vi "ModelDiscrimination.vi"() -> ()   [LabVIEW 2015]
uses:
  <vilib>/Platform/TimedLoop/XDataNode/timing_clust.ctl
  <vilib>/Platform/TimedLoop/XDataNode/nitl_modes.ctl
  <vilib>/Platform/TimedLoop/XDataNode/wakeup.ctl
  <vilib>/DAQmx/read.llb/DAQmx Read (Analog DBL 1Chan 1Samp).vi
  <vilib>/DAQmx/read.llb/DAQmx Read (Analog 1D DBL NChan 1Samp).vi
  <vilib>/DAQmx/create/channels.llb/DAQmx Create Channel (AI-Voltage-Basic).vi
  <vilib>/Enthought/Python Integration Toolkit/api/Unpack Double.vi
  <vilib>/DAQmx/miscellaneous.llb/DAQmx Fill In Error Info.vi
  <vilib>/Platform/TimedLoop/XDataNode/XDataNode.xnode
  Program Files/neMESYS_SDK/neMESYS LabVIEW Kit/neMESYS LabVIEW Integration Kit.lvlib
  <vilib>/Platform/TimedLoop/XDataNode/XDNodeRunTimeDep.lvlib
  Conor/Temp CN7500/Omega CN7500/Omega CN7500.lvlib
  <vilib>/Enthought/Python Integration Toolkit/Python Integration Toolkit.lvlib
panel:
  out "Record filename, RecordAmbInitisileFactorial1":string
  out "HPLC file name, MBDoE2peakin1":string
  out "Exp 9":bool
  out "Temp 9":dbl
  out "Flow 9":dbl
  out "Conc 9":dbl
  out "X2 A 8":dbl
  out "X2 ref A 8":dbl
  out "X2 B 8":dbl
  out "X ref B 8":dbl
  out "C BAcid 8":dbl
  out "C EB 8":dbl
  out "Exp 8":bool
  out "Temp 8":dbl
  out "Flow 8":dbl
  out "Conc 8":dbl
  out "X2 A 7":dbl
  out "X2 ref A 7":dbl
  out "X2 B 7":dbl
  out "X ref B 7":dbl
  out "C BAcid 7":dbl
  out "C EB 7":dbl
  out "Exp 7":bool
  out "Temp 7":dbl
  out "Flow 7":dbl
  out "Conc 7":dbl
  out "X2 A 6":dbl
  out "X2 ref A 6":dbl
  out "X2 B 6":dbl
  out "X ref B 6":dbl
  out "C BAcid 6":dbl
  out "C EB 6":dbl
  out "Exp 6":bool
  out "Temp 6":dbl
  out "Flow 6":dbl
  out "Conc 6":dbl
  out "X2 A 5":dbl
  out "X2 ref A 5":dbl
  out "X2 B 5":dbl
  out "X ref B 5":dbl
  out "C BAcid 5":dbl
  out "C EB 5":dbl
  out "Exp 5":bool
  out "Temp 5":dbl
  out "Flow 5":dbl
  out "Conc 5":dbl
  out "X2 A 4":dbl
  out "X2 ref A 4":dbl
  out "X2 B 4":dbl
  out "X ref B 4":dbl
  out "C BAcid 4":dbl
  out "C EB 4":dbl
  out "Exp 4":bool
  out "Temp 4":dbl
  out "Flow 4":dbl
  out "Conc 4":dbl
  out "X2 A 3":dbl
  out "X2 ref A 3":dbl
  out "X2 B 3":dbl
  out "X ref B 3":dbl
  out "C BAcid 3":dbl
  out "C EB 3":dbl
  out "Exp 3":bool
  out "Temp 3":dbl
  out "Flow 3":dbl
  out "Conc 3":dbl
  out "X2 A 2":dbl
  out "X2 ref A 2":dbl
  out "X2 B 2":dbl
  out "X ref B 2":dbl
  out "C BAcid 2":dbl
  out "C EB 2":dbl
  in  "Cat Mass (0.096 g)":dbl
  in  "Cat Diameter (825 um)":dbl
  out "X2 A 1":dbl
  out "X2 ref A 1":dbl
  out "X2 B 1":dbl
  out "X ref B 1":dbl
  out "Exp 1":bool
  out "C EB 1":dbl
  out "C BAcid 1":dbl
  out "Liquid Inlet Pressure (bar g)":dbl
  in  "Liquid P sensor Terminal Configuration":i32(ring)=-1 items=["default"=-1, "RSE"=10083, "NRSE"=10078, "Differential"=10106, "Pseudodifferential"=12529]
  in  "Liquid P sensor Physical Channel":tag="Dev1/ai0"
  out "Exp 2":bool
  out "Exp 0":bool
  out "Conc 1":dbl
  out "Flow 1":dbl
  out "Temp 1":dbl
  out "Conc 2":dbl
  out "Flow 2":dbl
  out "Temp 2":dbl
  out "X2 A":dbl
  out "X2 ref  A":dbl
  out "X2 B":dbl
  out "X2 ref B":dbl
  out "Desired Conc Not Possible":bool
  in  "Safety or Emergency Syringe Control":bool
  out "Feed Concentration (M)":dbl
  out "Total Flowrate (uL/min)":dbl
  out "Gas Back Pressure (barg)":dbl
  in  "Shut down in empty?\nLeft off, right on":bool
  in  "Clear":bool
  out "Safety Shut Down Pressure (barg)":dbl
  out "Calculated Pressure":dbl[](graph)
  out "Safety Shut Down Temp":dbl
  out "Actual Temp (oC)":dbl
  out "Temperature":dynamicdata(graph)
  out "Temp Set Point (oC)":dbl
  in  "Temp 0":dbl
  in  "Update Temperature Set Point":bool
  in  "Automated Experiments or Direct Control":bool
  in  "Set Point (oC)":dbl
  out "loop ind":dbl
  in  "Stop everything":bool
  in  "Skip Exp":bool
  in  "Minutes between Exp":dbl min=0.0 step=0.05
  in  "Refill 4":bool
  in  "Refill 3":bool
  in  "Refill 2":bool
  in  "Refill 1":bool
  in  "Empty 4":bool
  in  "Empty 3":bool
  in  "Empty 2":bool
  in  "Empty 1":bool
  in  "Calibrate 4":bool
  in  "Calibrate 3":bool
  in  "Calibrate 2":bool
  in  "Calibrate 1":bool
  in  "Stop Dose 4":bool
  in  "Stop Dose 3":bool
  in  "Stop Dose 2":bool
  in  "Stop Dose 1":bool
  in  "Flow 0":dbl
  in  "Conc 0":dbl
  in  "Generate Flow":bool
  in  "Set Flowrate 1":dbl
  in  "Set Flowrate 2":dbl
  in  "Set Flowrate 3":dbl
  in  "Set Flowrate 4":dbl
  in  "High Conc":dbl min=0.0 max=2.0
  in  "Low Conc":dbl min=0.0 max=2.0
  out "Syringe Level 4":dbl(slide) scale=0.0..5500.0
  out "Syringe Level 3":dbl(slide) scale=0.0..5500.0
  out "Syringe Level 2":dbl(slide) scale=0.0..5500.0
  out "Syringe Level 1":dbl(slide) scale=0.0..5500.0
  out "Flowrate 4 High":dbl
  out "Flowrate 3 High":dbl
  out "Flowrate 2 Low":dbl
  out "Flowrate 1 Low":dbl
  # "Pre Planned Experiments"
  # "Conducted Experiments Set Points"
  # "Safety (start and end)"
  # "Current Conditions"
  # "(uL/min)"
  # "Coerced to nearest possible"
  # "Experimental Info"
  # "This code only does Automated \nDirect control just sets all variables to 0"
  # "Direct Control"
  # "Unit of Gas Flow NmL/min"
  # "Emergency Syringe Control Below"
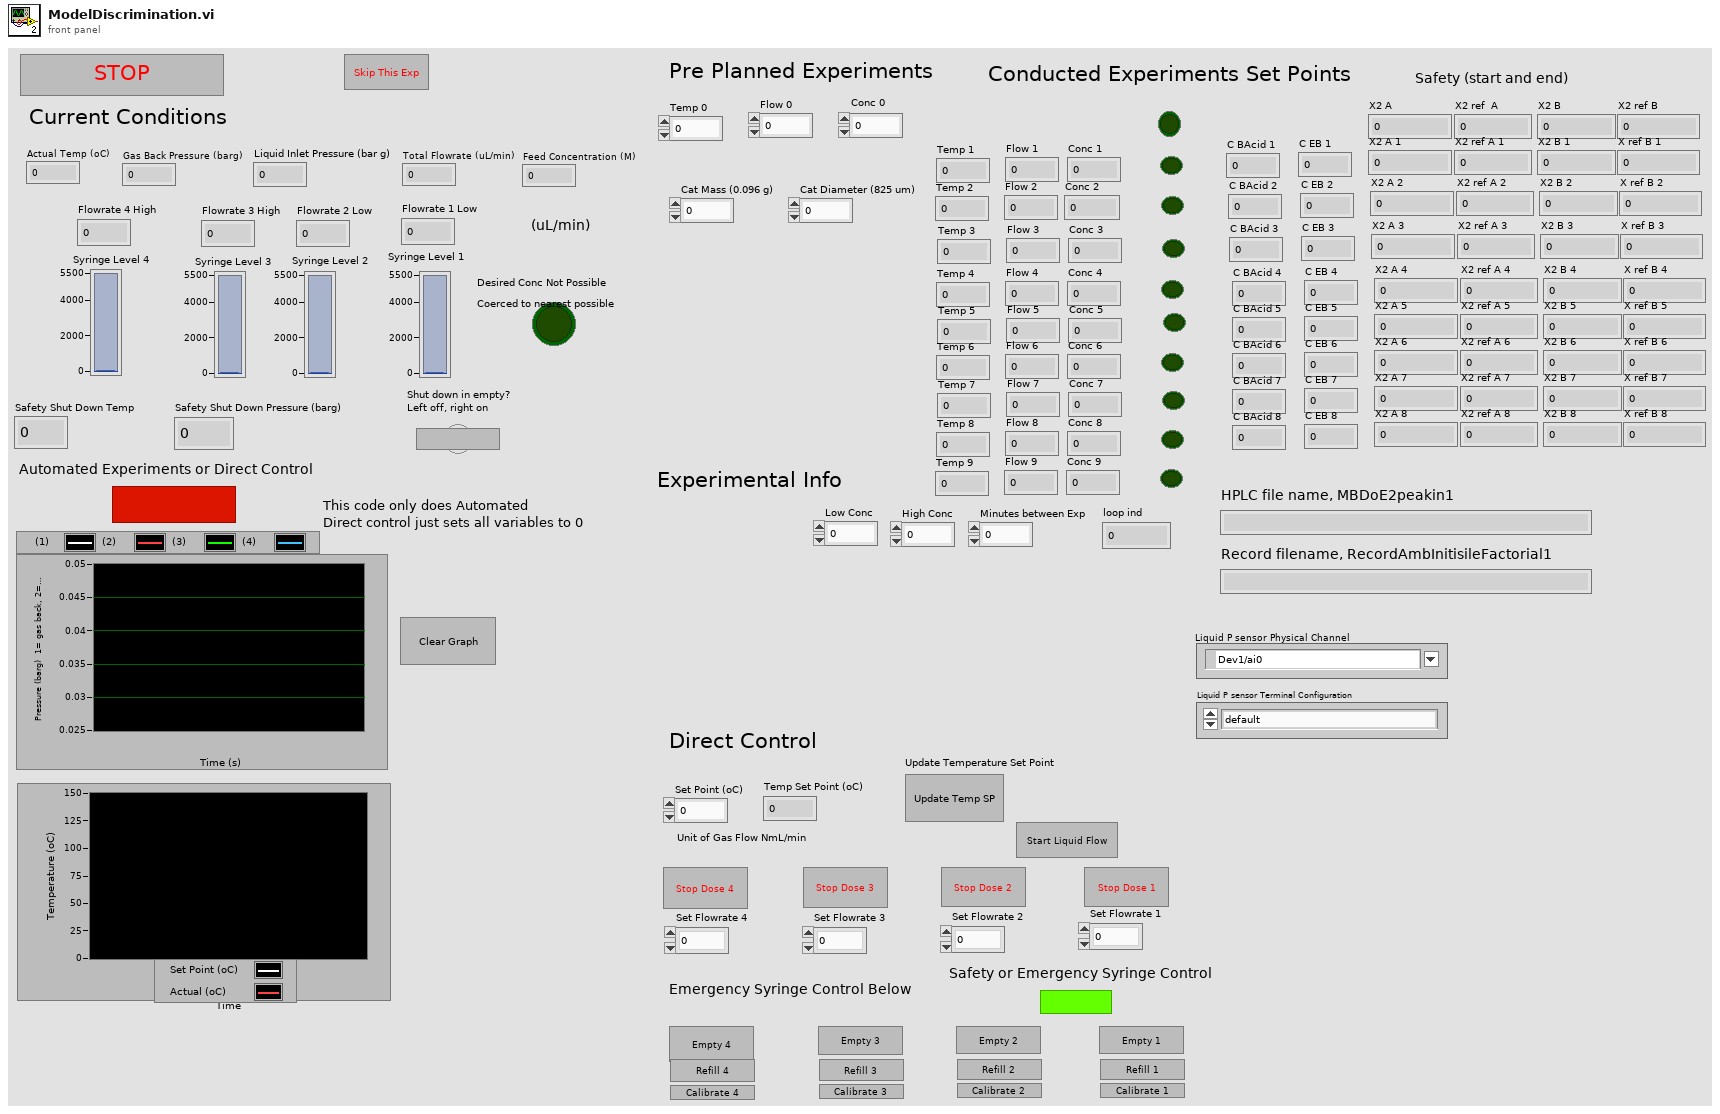
[diagram p1: front panel]
types:
  T1 = typedef "XDNodeRunTimeDep.lvlib/timing_clust.ctl" = cluster{"Expected End [f-1]":u64, "Actual End [f-1]":u64, "Finished Late? [f-1]":bool, "Expected End [i-1]":u64, "Actual End [i-1]":u64, "Finished Late? [i-1]":bool, "Expected Start [i]":u64, "Actual Start [i]":u64, "Expected Start [f]":u64, "Actual Start [f]":u64, "Source Name":string, "Structure Name":string, "Period":i64, "Deadline":i64, "Offset":i64, "Start":i64, "Priority":i32, "Timeout":i32, "Mode":T2, "Wakeup Reason":T3, "Error":errorcluster, "Source Type":string, "Secondary Source Type":string, "Global End Time":u64, "Global Start Time":u64, "Frame Duration":u64, "Iteration Duration":u64, "Assigned CPU":i32, "I/O Scan Engine Mode":u32}
  T2 = typedef "XDNodeRunTimeDep.lvlib/nitl_modes.ctl" = enum32{"No Change", "Process missed periods, maintain original phase", "Discard missed periods, maintain original phase", "Process missed periods, ignore original phase", "Discard missed periods, ignore original phase"}
  T3 = typedef "XDNodeRunTimeDep.lvlib/wakeup.ctl" = enum32{"Normal", "Aborted", "Asynchronous wakeup", "Timing source error", "Timed loop error", "Timeout"}
  T4 = typedef "Python Integration Toolkit.lvlib/Session ID.ctl" = u64
  T5 = typedef "Python Integration Toolkit.lvlib/Python Objects.ctl" = variant
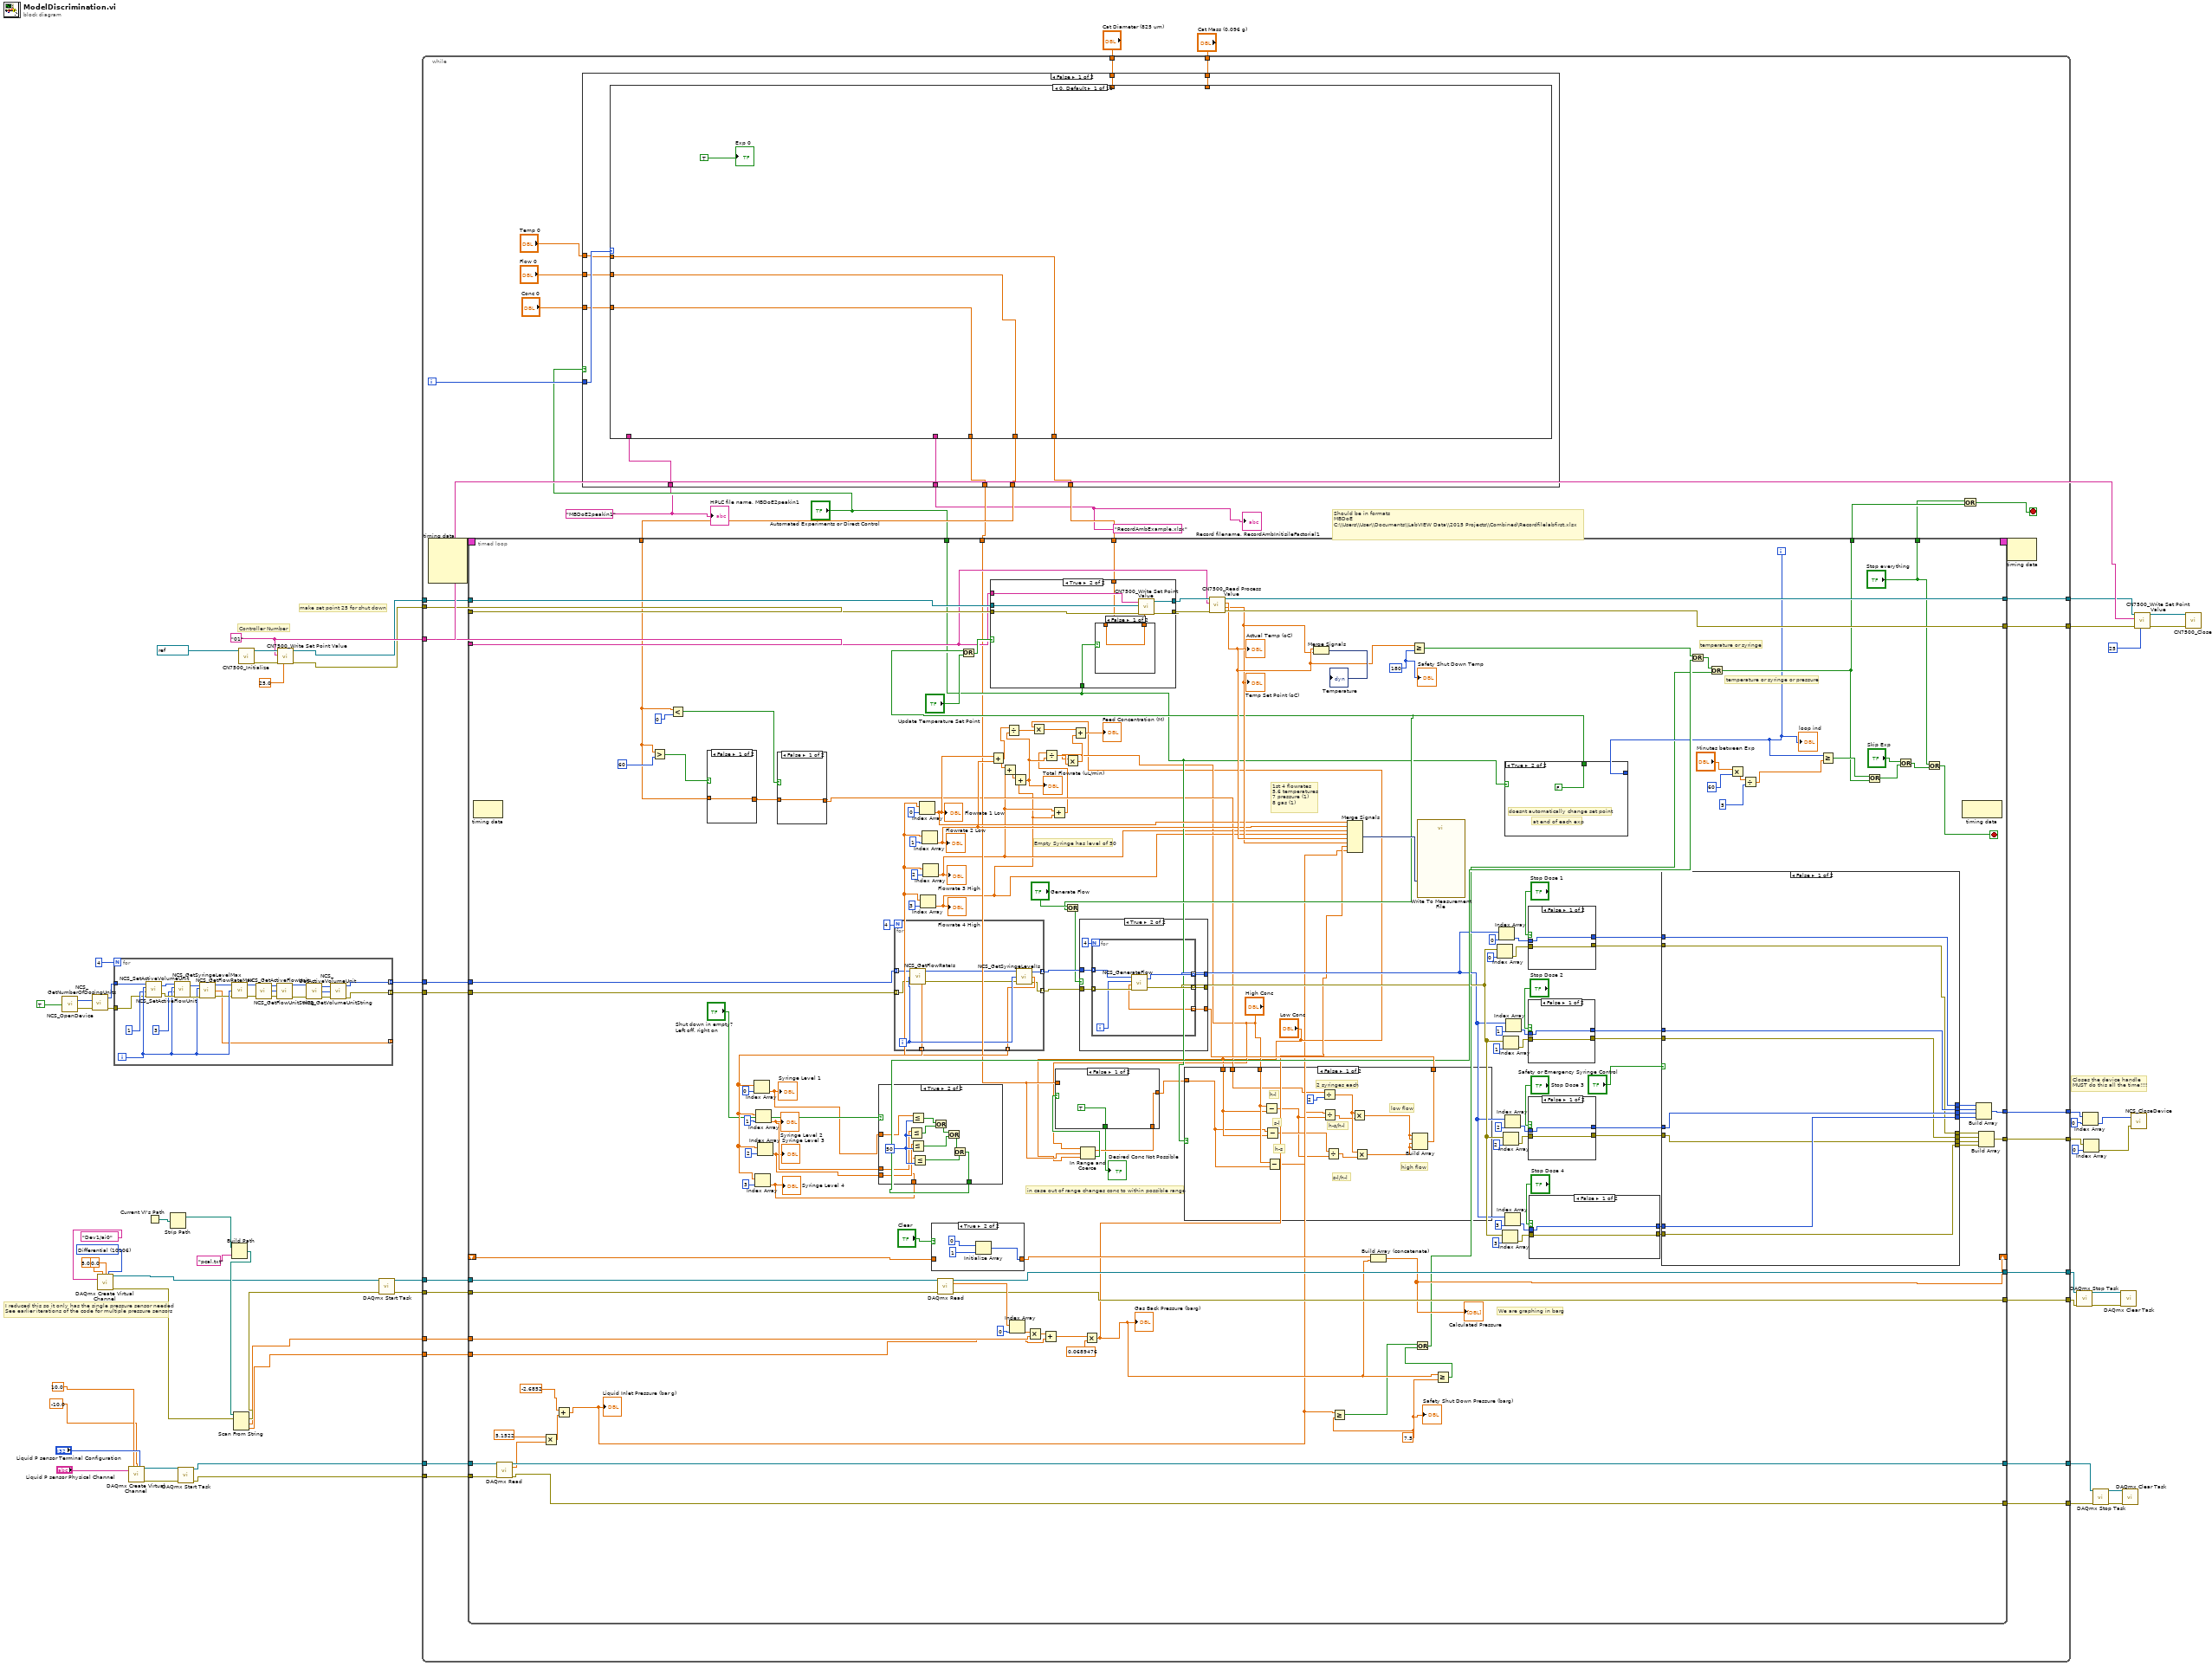
[diagram p0: block diagram]
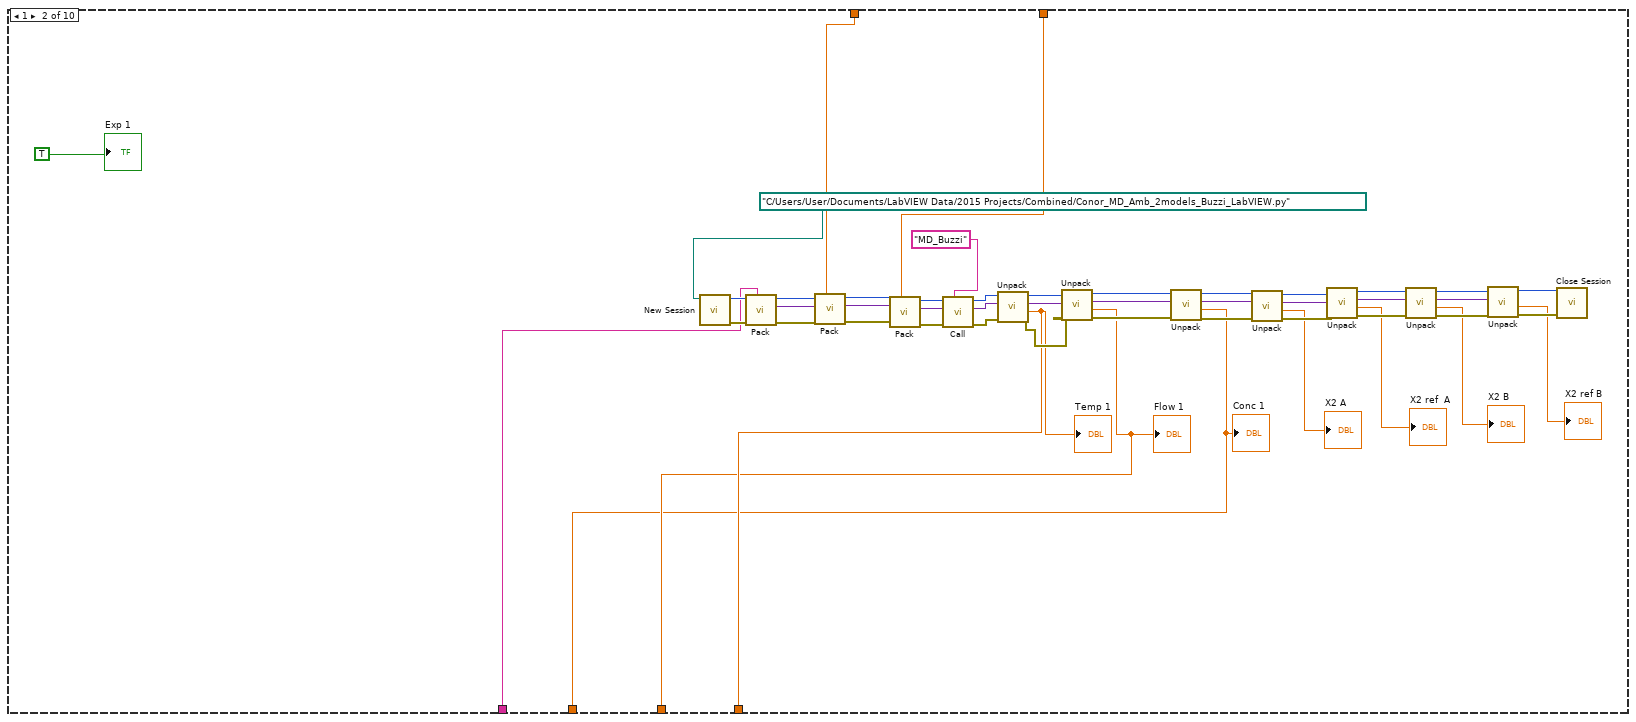
[diagram p2: hidden frame]
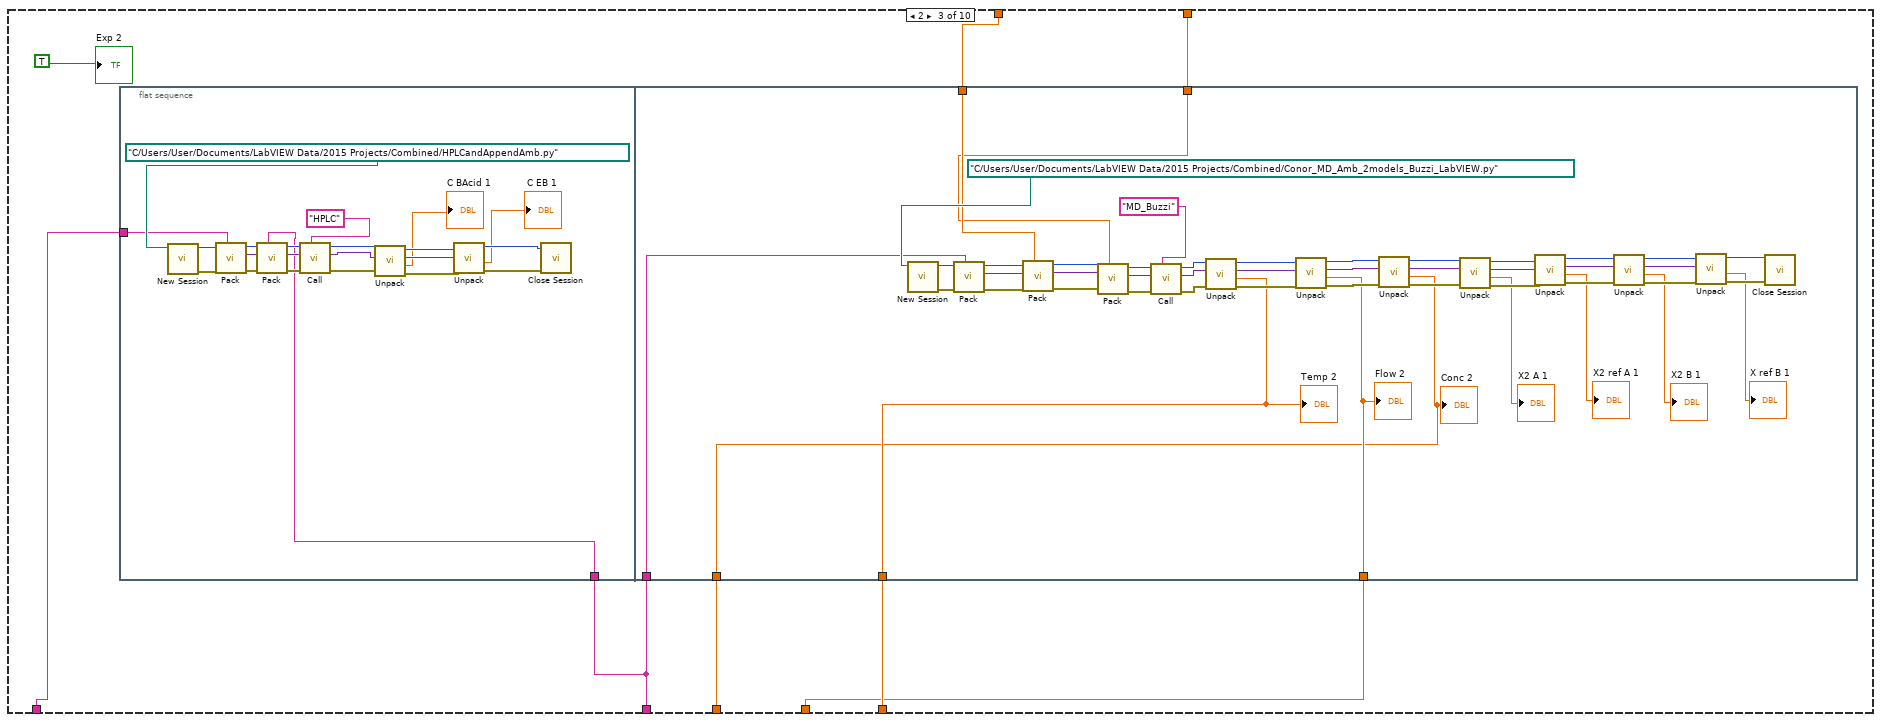
[diagram p3: hidden frame]
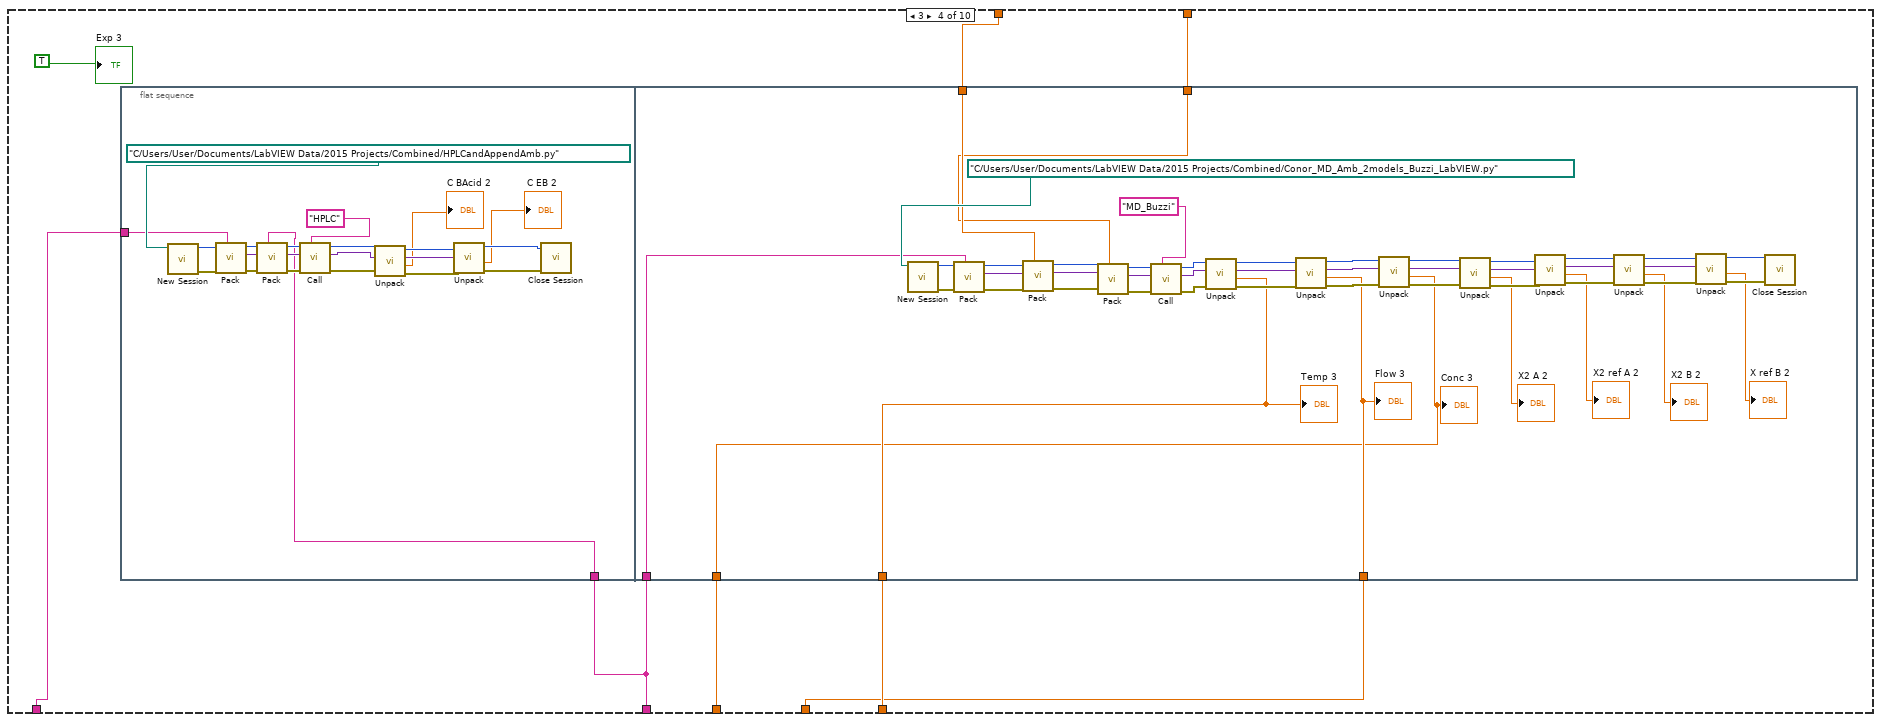
[diagram p4: hidden frame]
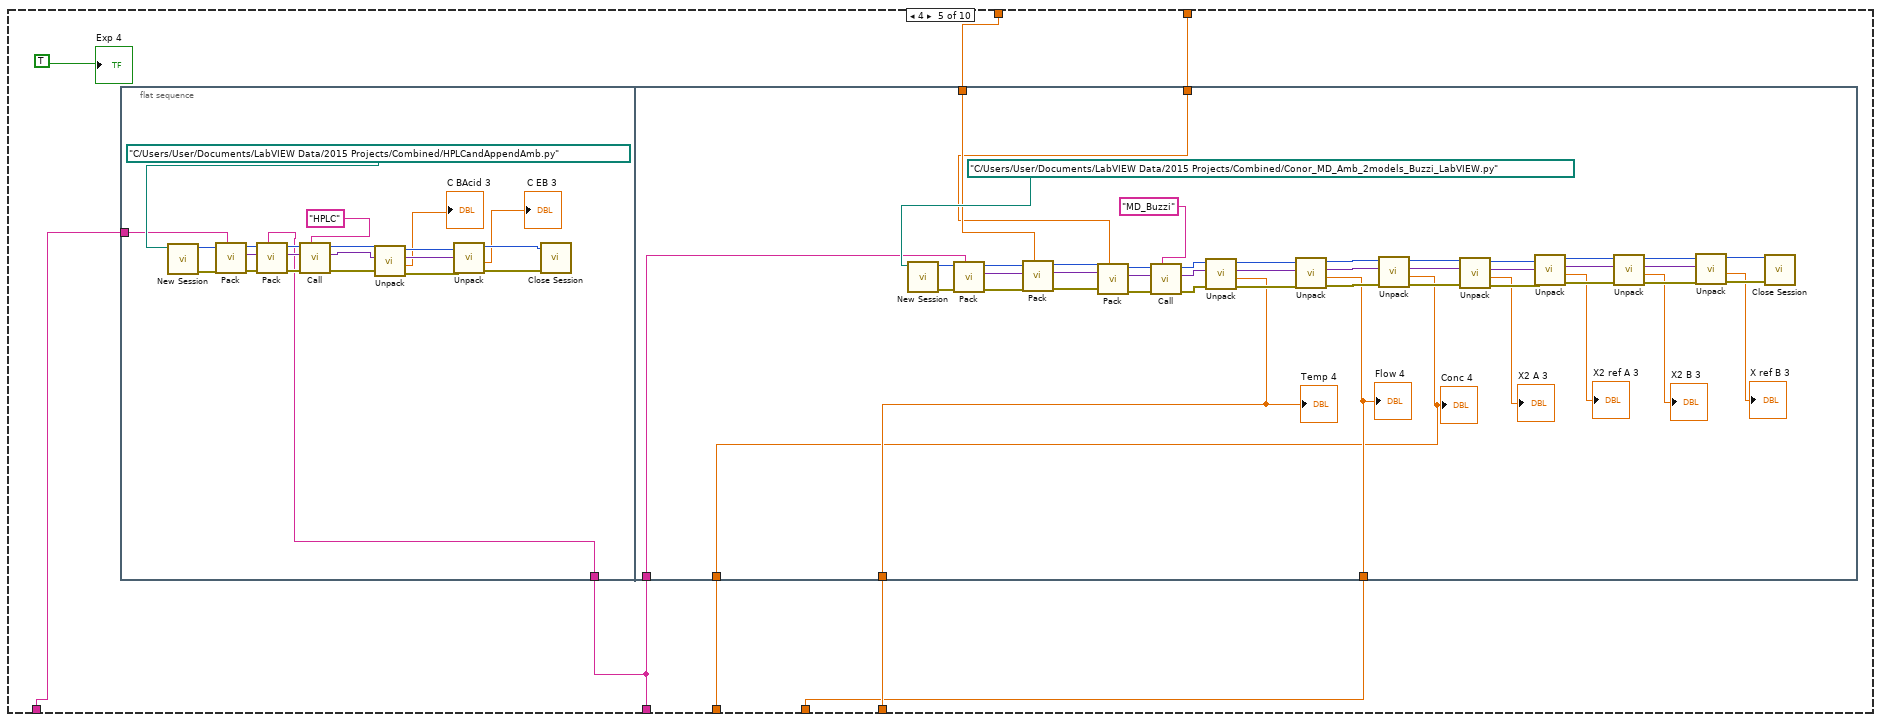
[diagram p5: hidden frame]
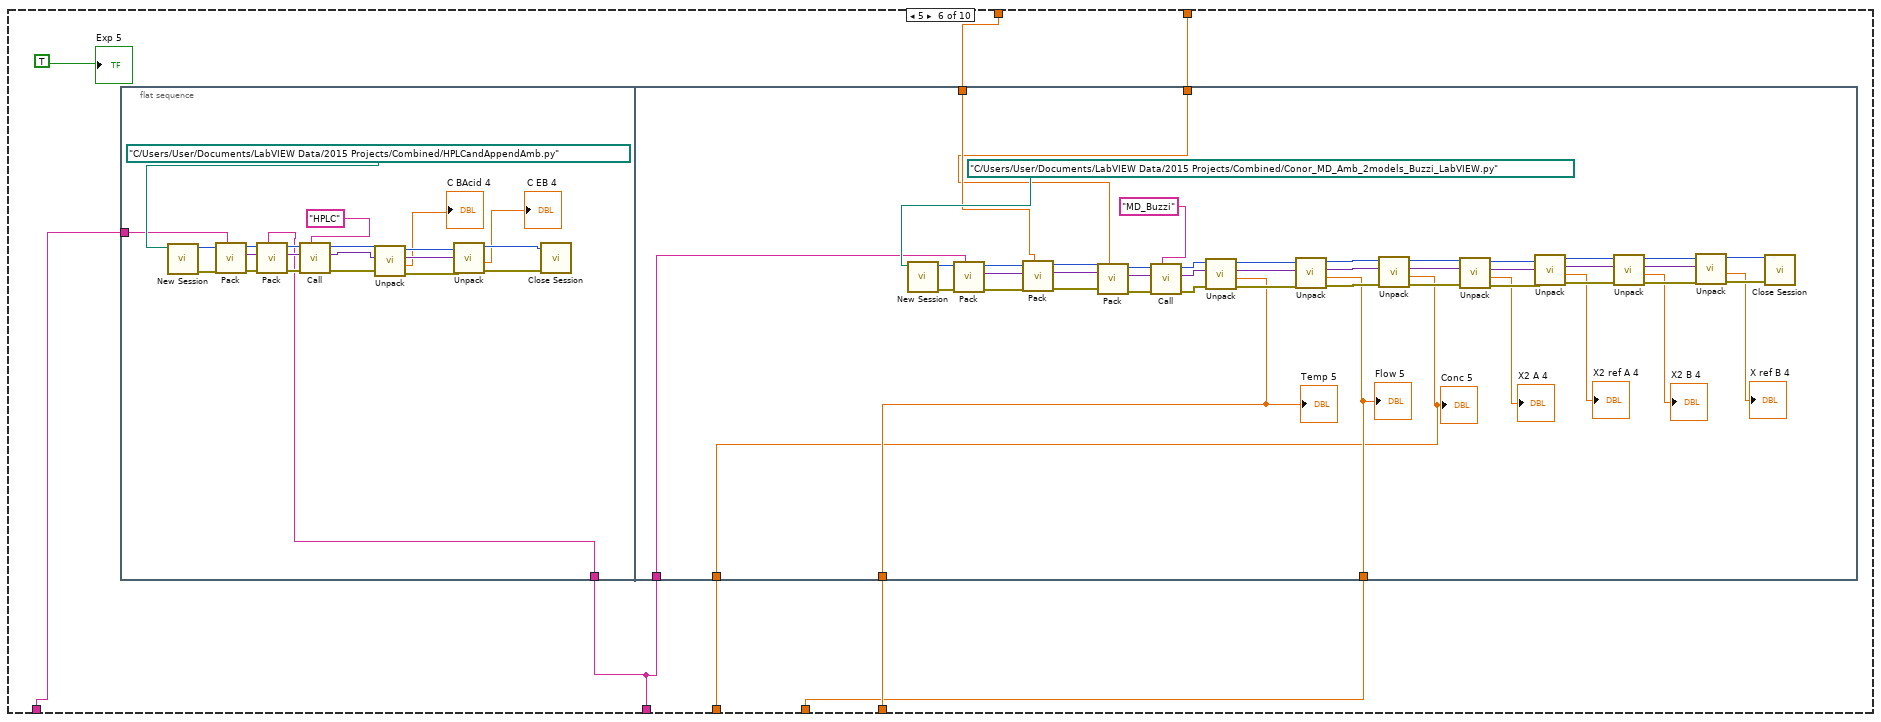
[diagram p6: hidden frame]
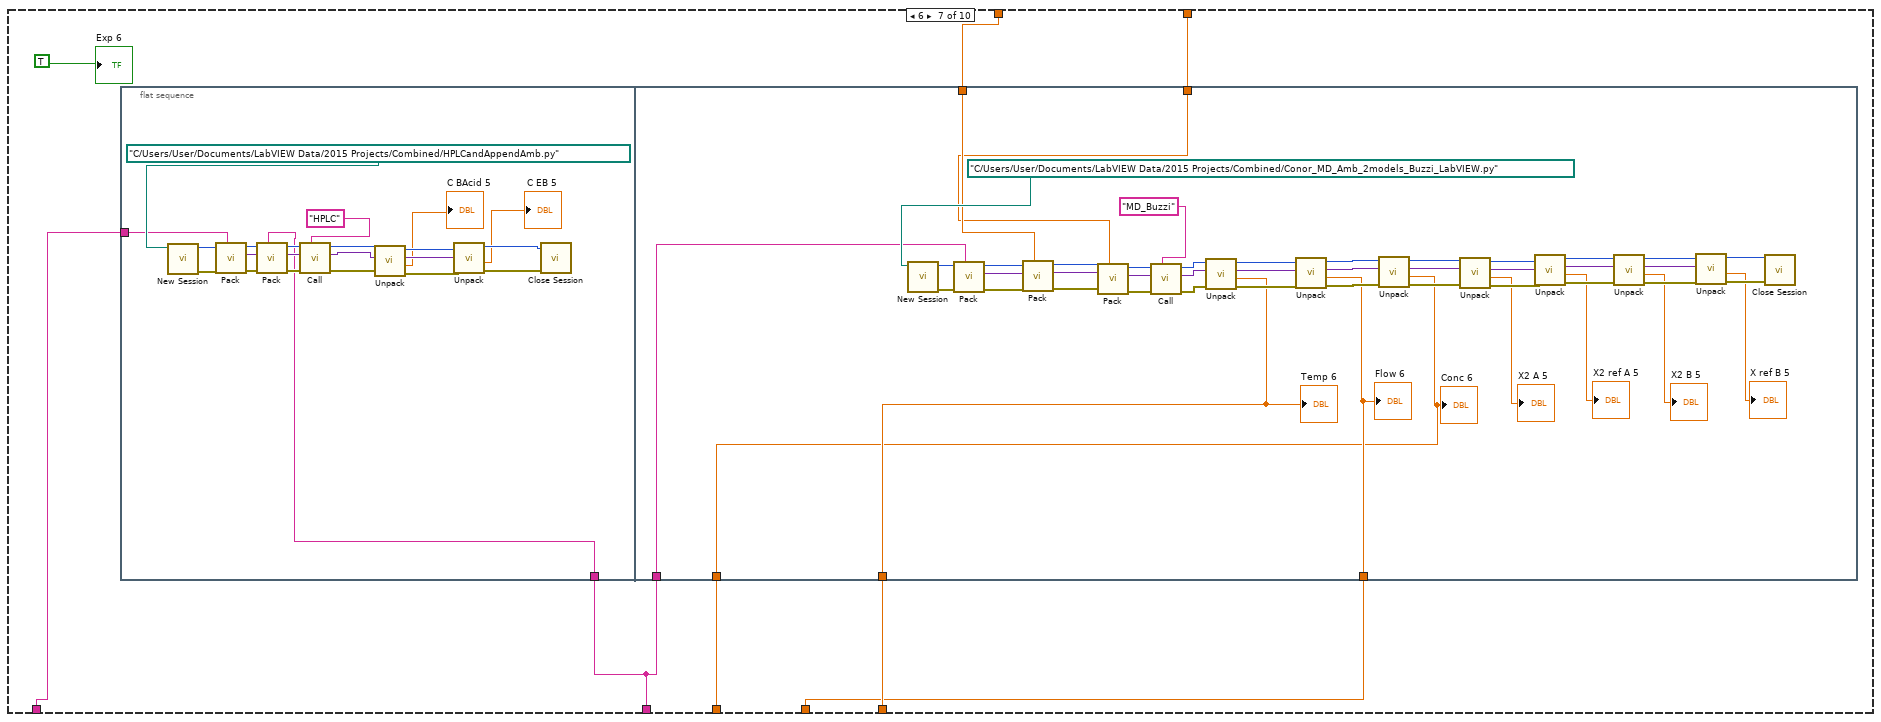
[diagram p7: hidden frame]
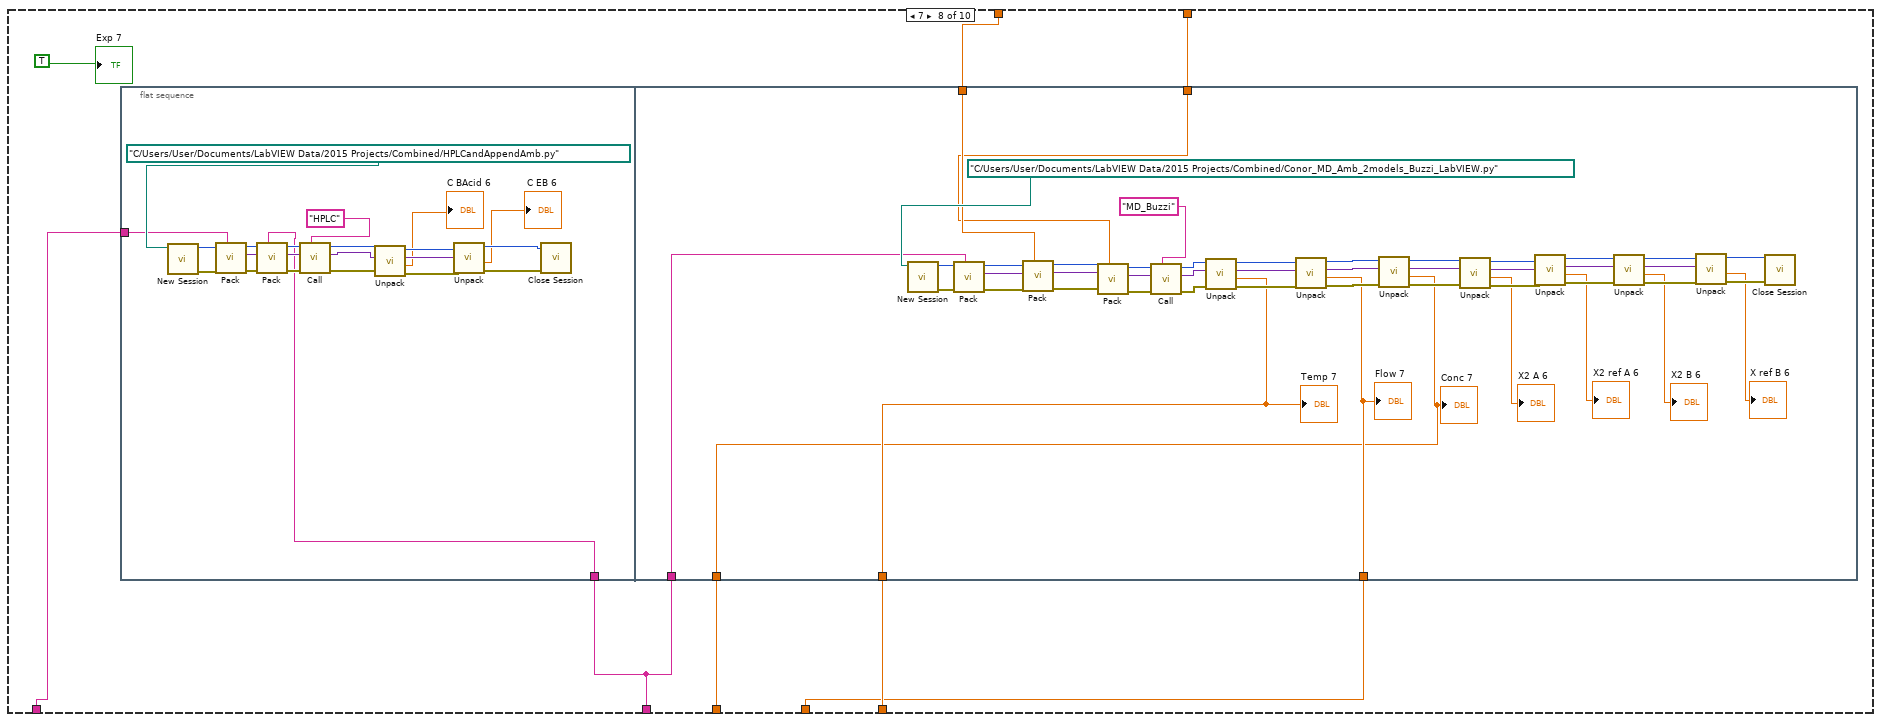
[diagram p8: hidden frame]
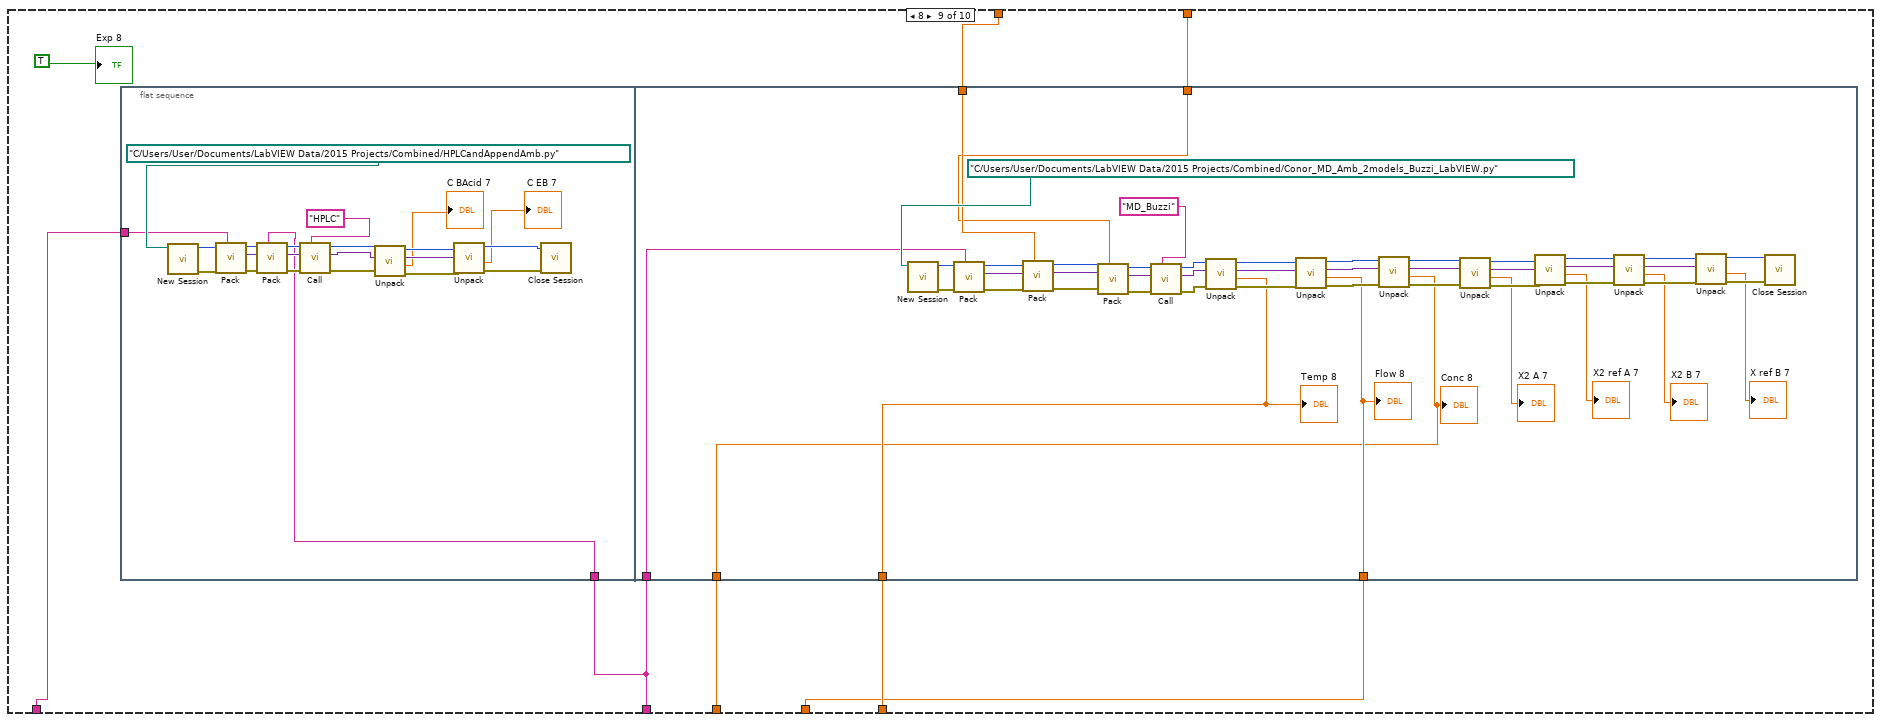
[diagram p9: hidden frame]
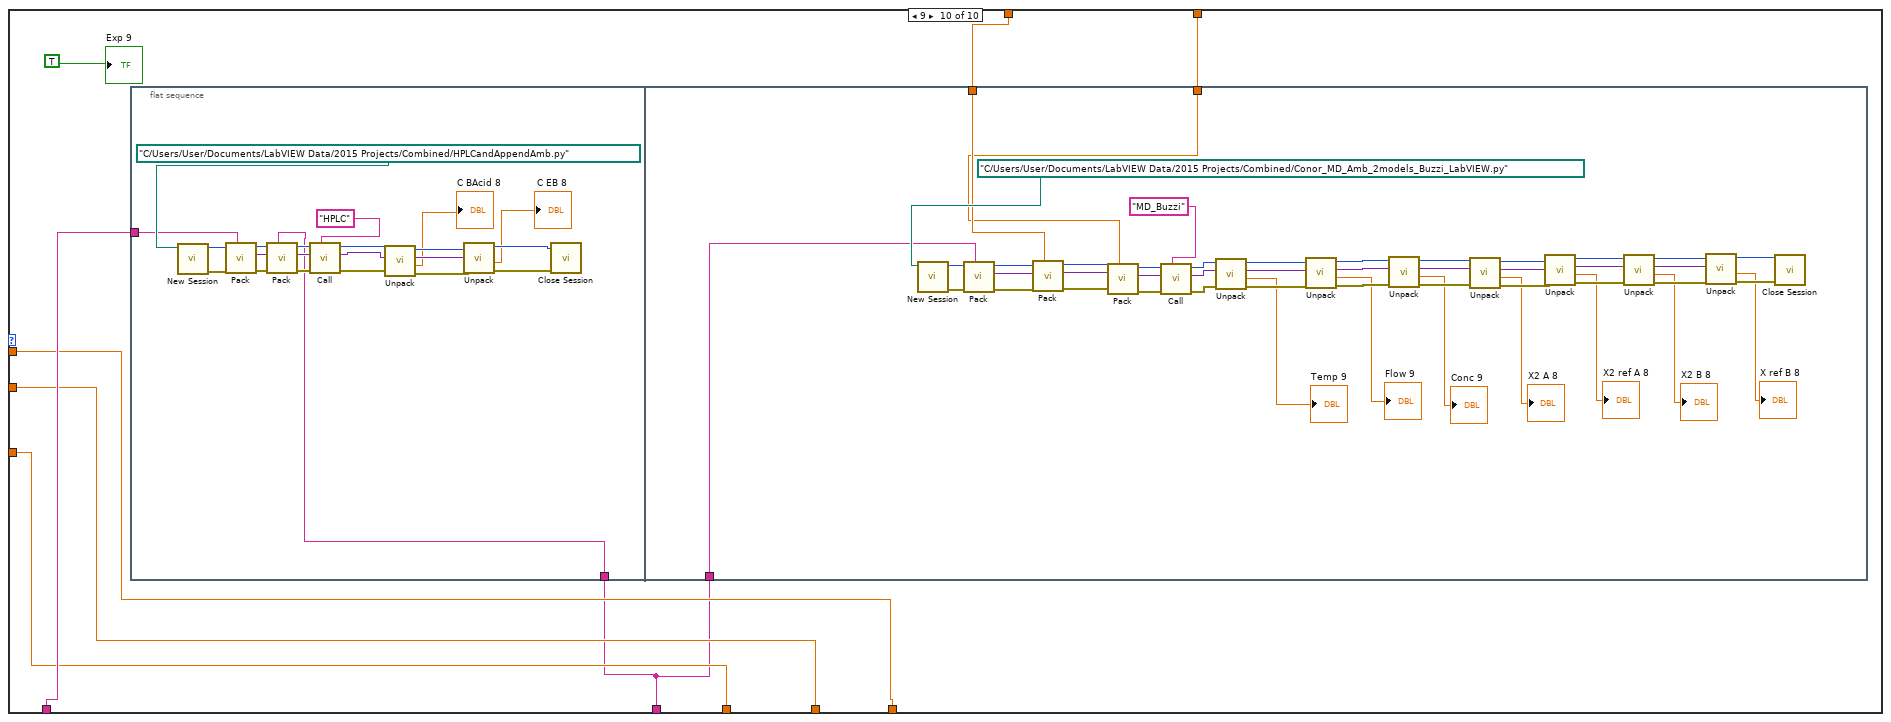
[diagram p10: hidden frame]
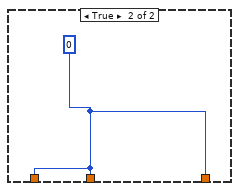
[diagram p11: hidden frame]
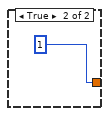
[diagram p12: hidden frame]
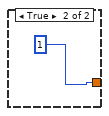
[diagram p13: hidden frame]
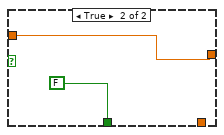
[diagram p14: hidden frame]
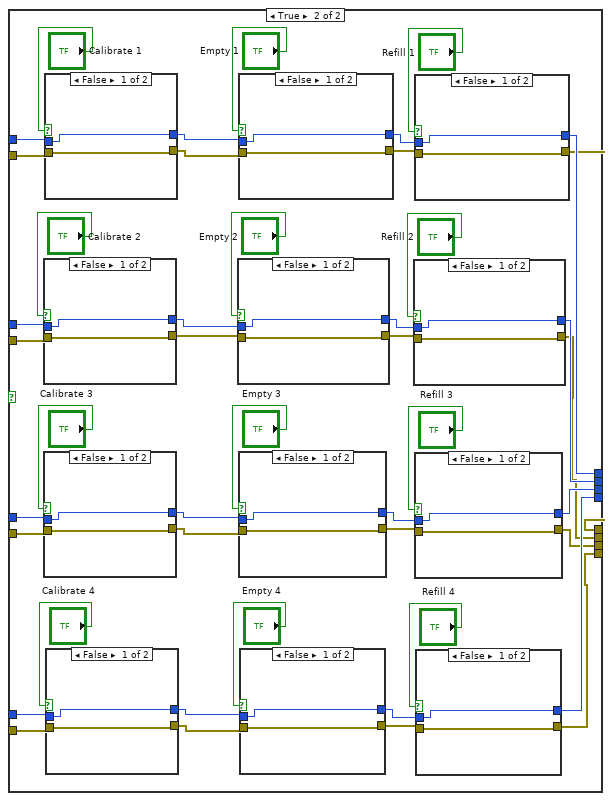
[diagram p15: hidden frame]
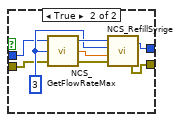
[diagram p16: hidden frame]
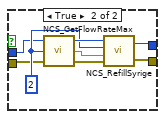
[diagram p17: hidden frame]
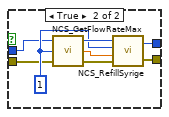
[diagram p18: hidden frame]
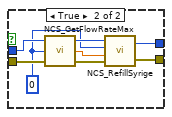
[diagram p19: hidden frame]
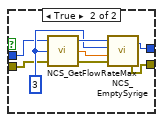
[diagram p20: hidden frame]
diagram:
  w31 = 10106 items=["default"=-1, "RSE"=10083, "NRSE"=10078, "Differential"=10106, "Pseudodifferential"=12529] ("input terminal configuration")
  w38 = "01" ("Controller Number")
  # "I reduced this so it only has the single pressure sensor needed\nSee earlier iterations of the code for multiple pressure sensors"
  # "make set point 25 for shut down"
  # "Controller Number"
  # "Closes the device handle \nMUST do this all the time!!!!"
  n1 = call "NCS_OpenDevice.vi"("show status window"=TRUE) -> ("device handle"=w57:u32, "error out"=w56:errorcluster)
  n2 = call "NCS_GetNumberOfDosingUnits.vi"("device handle in"=w57, "error in (no error)"=w56) -> ("device handle out"=w54:u32, "error out"=w55:errorcluster)  [unwired: 1 out]
  n3 = call-poly <vilib>:"DAQmx Create Virtual Channel.vi"("maximum value"=5.0, "minimum value"=0.0, "input terminal configuration"=w31, "physical channels"=tag "Dev1/ai0") -> ("task out"=w15:refnum<k21>, "error out"=w16:errorcluster)  [unwired: 10 in]
  n4 = for {
    N: 4 -> [_]
    tunnel: [w63] -> w53 mode=indexing
    tunnel: [w62] -> w52 mode=indexing
    tunnel: [w76] -> _ mode=indexing
    tunnel: w55 -> [w61]
    tunnel: w54 -> [w60]
    i -> [w79]
    n5 = call "NCS_SetActiveVolumeUnit.vi"("error in (no error)"=w61, "active volume unit"=1, "dosingunit"=w79, "device handle in"=w60) -> ("error out"=w82:errorcluster, "device handle out"=w83:u32)
    n6 = call "NCS_SetActiveFlowUnit.vi"("error in (no error)"=w82, "active flow unit"=3, "dosingunit"=w79, "device handle in"=w83) -> ("error out"=w80:errorcluster, "device handle out"=w81:u32)
    n7 = call "NCS_GetSyringeLevelMax.vi"("error in (no error)"=w80, "dosingunit"=w79, "device handle in"=w81) -> ("error out"=w77:errorcluster, "syringe level max"=w76:dbl, "device handle out"=w78:u32)  [unwired: 1 out]
    n8 = call "NCS_GetFlowRateMax.vi"("error in (no error)"=w77, "dosingunit"=w79, "device handle in"=w78) -> ("error out"=w64:errorcluster, "device handle out"=w65:u32)  [unwired: 1 out]
    n9 = call "NCS_GetActiveFlowUnit.vi"("error in (no error)"=w64, "device handle in"=w65) -> ("error out"=w72:errorcluster, "active flow unit"=w71:u8, "device handle out"=w73:u32)  [unwired: 1 in]
    n10 = call "NCS_GetFlowUnitString.vi"("device handle in"=w73, "flow unit id"=w71, "error in (no error)"=w72) -> ("device handle out"=w68:u32, "error out"=w67:errorcluster)  [unwired: 2 out]
    n11 = call "NCS_GetActiveVolumeUnit.vi"("error in (no error)"=w67, "device handle in"=w68) -> ("error out"=w69:errorcluster, "active volume unit"=w70:u8, "device handle out"=w66:u32)  [unwired: 1 in]
    n12 = call "NCS_GetVolumeUnitString.vi"("device handle in"=w66, "volume unit id"=w70, "error in (no error)"=w69) -> ("device handle out"=w63:u32, "error out"=w62:errorcluster)  [unwired: 2 out]
  }
  n13 = call-poly <vilib>:"DAQmx Create Virtual Channel.vi"("maximum value"=10.0, "minimum value"=-10.0 ("maximum value"), "input terminal configuration"="Liquid P sensor Terminal Configuration", "physical channels"="Liquid P sensor Physical Channel") -> ("task out"=w11:refnum<k21>, "error out"=w12:errorcluster)  [unwired: 10 in]
  n14 = Current VI's Path() -> (path=w29:path)
  n15 = Strip Path(path=w29) -> (stripped path=w27:path)  [unwired: 1 out]
  n16 = call <vilib>:"DAQmx Start Task.vi"("task/channels in"=w11, "error in"=w12) -> ("task out"=w10:refnum<k21>, "error out"=w9:errorcluster)  [unwired: 12 in]
  n17 = Build Path(base path=w27, name or relative path="pcal.txt") -> (appended path=w28:path)
  n18 = Scan From String(w28, w16) -> (w25:errorcluster, output 1=w22:dbl, output 2=w21:dbl)  [unwired: 3 in, 1 out]
  n19 = call "CN7500_Initialize.vi"("VISA resource name"=refnum<visa-resource-name> "COM8") -> ("error out"=w44:errorcluster, "VISA resource name out"=w45:refnum<visa-resource-name>)  [unwired: 9 in]
  n20 = call "CN7500_Write Set Point Value.vi"("Target Set Point Value"=25.0, "error in (no error)"=w44, "Controller Number"=w38, "VISA In"=w45) -> ("error out"=w36:errorcluster, "VISA Out"=w37:refnum<visa-resource-name>)  [unwired: 6 in]
  n21 = call <vilib>:"DAQmx Start Task.vi"("task/channels in"=w15, "error in"=w25) -> ("task out"=w24:refnum<k21>, "error out"=w23:errorcluster)  [unwired: 12 in]
  n22 = while {
    tunnel: w53 -> [w119]
    tunnel: w52 -> [w118]
    tunnel: [w117] -> w47
    tunnel: [w116] -> w46
    tunnel: w38 -> [w113]
    tunnel: w37 -> [w112]
    tunnel: w36 -> [w111]
    tunnel: [w110] -> w35
    tunnel: [w109] -> w34
    tunnel: w24 -> [w107]
    tunnel: w23 -> [w106]
    tunnel: w22 -> [w105]
    tunnel: w21 -> [w104]
    tunnel: [w103] -> w18
    tunnel: [w102] -> w17
    tunnel: w10 -> [w91]
    tunnel: w9 -> [w90]
    tunnel: [w89] -> w7
    tunnel: [w88] -> w5
    tunnel: "Cat Diameter (825 um)" -> [w87]
    tunnel: "Cat Mass (0.096 g)" -> [w86]
    i -> [w96]
    stop <- w101 stop-if-true
    w84 = "RecordAmbExample.xlsx" ("Result file name must end with .xlsx")
    w85 = "MBDoE2peakin1" ("HPLC file Name, dont need extension")
    # "Should be in formats \nMBDoE\nC:\\\\Users\\\\User\\\\Documents\\\\LabVIEW Data\\\\2015 Projects\\\\Combined\\Recordfilelabfirst.xlsx"
    n23 = node-c288() -> (w115:T1)  [unwired: 4 in]
    n24 = case shown="False" "Automated Experiments or Direct Control" {
      tunnel: [w127 w790] -> w99
      tunnel: [w125 w790] -> w98
      tunnel: [w129 w790] -> w97
      tunnel: w96 -> [w130 _]
      tunnel: "Conc 0" -> [w128 _]
      tunnel: "Flow 0" -> [w124 _]
      tunnel: "Temp 0" -> [w126 _]
      tunnel: w85 -> [w122 _]
      tunnel: w84 -> [w123 _]
      tunnel: w87 -> [w121 _]
      tunnel: w86 -> [w120 _]
      frame False {
        n25 = case shown="0, Default" w130 {
          tunnel: [w132 w135 w185 w261 w337 w413 w489 w565 w641 w717] -> w129
          tunnel: w128 -> [w132 _ _ _ _ _ _ _ _ w717]
          tunnel: [w134 w137 w187 w263 w339 w415 w491 w567 w643 w719] -> w127
          tunnel: w126 -> [w134 _ _ _ _ _ _ _ _ w719]
          tunnel: [w133 w136 w186 w262 w338 w414 w490 w566 w642 w718] -> w125
          tunnel: w124 -> [w133 _ _ _ _ _ _ _ _ w718]
          tunnel: w123 -> [_ w142 w184 w260 w336 w412 w488 w564 w640 w716]
          tunnel: w122 -> [_ _ w188 w264 w340 w416 w492 w568 w644 w720]
          tunnel: w121 -> [_ w145 w183 w259 w335 w411 w487 w563 w639 w715]
          tunnel: w120 -> [_ w144 w182 w258 w334 w410 w486 w562 w638 w714]
          frame 0, Default {
            "Exp 0" <- TRUE
          }
          frame 1 {
            n26 = call <vilib>:"New Session.vi"("Path to Python Module (.py File)"=path "C:/Users/User/Documents/LabVIEW Data/2015 Projects/Combined/Conor_MD_Amb_2models_Buzzi_LabVIEW.py") -> ("error out"=w173:errorcluster, "Session ID out"=w172:T4)  [unwired: 9 in]
            n27 = call <vilib>:"Pack.vi"("Argument"=w142, "error in (no error)"=w173, "Session ID"=w172) -> ("error out"=w166:errorcluster, "Python Object References Out"=w167:T5, "Session ID out"=w168:T4)  [unwired: 6 in]
            n28 = call <vilib>:"Pack.vi"("Argument"=w145, "error in (no error)"=w166, "Python Object References In"=w167, "Session ID"=w168) -> ("error out"=w148:errorcluster, "Python Object References Out"=w150:T5, "Session ID out"=w149:T4)  [unwired: 5 in]
            n29 = call <vilib>:"Pack.vi"("Argument"=w144, "error in (no error)"=w148, "Python Object References In"=w150, "Session ID"=w149) -> ("error out"=w151:errorcluster, "Python Object References Out"=w152:T5, "Session ID out"=w153:T4)  [unwired: 5 in]
            n30 = call <vilib>:"Call.vi"("Function or Method Name"="MD_Buzzi", "error in (no error)"=w151, "Python Object References In"=w152, "Session ID"=w153) -> ("error out"=w159:errorcluster, "Python Object References Out"=w162:T5, "Session ID out"=w165:T4)  [unwired: 5 in]
            n31 = call-poly <vilib>:"Unpack.vi"("error in (no error)"=w159, "Python Object References In"=w162, "Session ID"=w165) -> ("error out"=w158:errorcluster, "Value"=w137:dbl, "Python Object References Out"=w161:T5, "Session ID out"=w164:T4)  [unwired: 5 in]
            "Temp 1" <- w137
            n32 = call-poly <vilib>:"Unpack.vi"("error in (no error)"=w158, "Python Object References In"=w161, "Session ID"=w164) -> ("error out"=w157:errorcluster, "Value"=w136:dbl, "Python Object References Out"=w160:T5, "Session ID out"=w163:T4)  [unwired: 5 in]
            "Flow 1" <- w136
            n33 = call-poly <vilib>:"Unpack.vi"("error in (no error)"=w157, "Python Object References In"=w160, "Session ID"=w163) -> ("error out"=w154:errorcluster, "Value"=w135:dbl, "Python Object References Out"=w155:T5, "Session ID out"=w156:T4)  [unwired: 5 in]
            "Conc 1" <- w135
            n34 = call-poly <vilib>:"Unpack.vi"("error in (no error)"=w154, "Python Object References In"=w155, "Session ID"=w156) -> ("error out"=w178:errorcluster, "Value"=→"X2 A":dbl, "Python Object References Out"=w176:T5, "Session ID out"=w174:T4)  [unwired: 5 in]
            n35 = call-poly <vilib>:"Unpack.vi"("error in (no error)"=w178, "Python Object References In"=w176, "Session ID"=w174) -> ("error out"=w179:errorcluster, "Value"=→"X2 ref  A":dbl, "Python Object References Out"=w177:T5, "Session ID out"=w175:T4)  [unwired: 5 in]
            n36 = call-poly <vilib>:"Unpack.vi"("error in (no error)"=w179, "Python Object References In"=w177, "Session ID"=w175) -> ("error out"=w180:errorcluster, "Value"=→"X2 B":dbl, "Python Object References Out"=w171:T5, "Session ID out"=w170:T4)  [unwired: 5 in]
            n37 = call-poly <vilib>:"Unpack.vi"("error in (no error)"=w180, "Python Object References In"=w171, "Session ID"=w170) -> ("error out"=w146:errorcluster, "Value"=→"X2 ref B":dbl, "Session ID out"=w147:T4)  [unwired: 5 in, 1 out]
            n38 = call <vilib>:"Close Session.vi"("error in (no error)"=w146, "Session ID"=w147) -> ()  [unwired: 9 in, 1 out]
            "Exp 1" <- TRUE
          }
          frame 2 {
            n39 = flat-sequence {
              tunnel: w188 -> [w199]
              tunnel: w184 -> [w192]
              tunnel: [w221] -> w187
              tunnel: [w220] -> w186
              tunnel: [w219] -> w185
              tunnel: w184 -> [w214]
              tunnel: w183 -> [w213]
              tunnel: w182 -> [w212]
              frame #0 {
                n40 = call <vilib>:"New Session.vi"("Path to Python Module (.py File)"=path "C:/Users/User/Documents/LabVIEW Data/2015 Projects/Combined/HPLCandAppendAmb.py") -> ("error out"=w208:errorcluster, "Session ID out"=w207:T4)  [unwired: 9 in]
                n41 = call <vilib>:"Pack.vi"("Argument"=w199, "error in (no error)"=w208, "Session ID"=w207) -> ("error out"=w194:errorcluster, "Python Object References Out"=w196:T5, "Session ID out"=w198:T4)  [unwired: 6 in]
                n42 = call <vilib>:"Pack.vi"("Argument"=w192, "error in (no error)"=w194, "Python Object References In"=w196, "Session ID"=w198) -> ("error out"=w193:errorcluster, "Python Object References Out"=w195:T5, "Session ID out"=w197:T4)  [unwired: 5 in]
                n43 = call <vilib>:"Call.vi"("Function or Method Name"="HPLC", "error in (no error)"=w193, "Python Object References In"=w195, "Session ID"=w197) -> ("error out"=w209:errorcluster, "Python Object References Out"=w200:T5, "Session ID out"=w201:T4)  [unwired: 5 in]
                n44 = call-poly <vilib>:"Unpack.vi"("error in (no error)"=w209, "Python Object References In"=w200, "Session ID"=w201) -> ("error out"=w210:errorcluster, "Value"=→"C BAcid 1":dbl, "Python Object References Out"=w205:T5, "Session ID out"=w204:T4)  [unwired: 5 in]
                n45 = call-poly <vilib>:"Unpack.vi"("error in (no error)"=w210, "Python Object References In"=w205, "Session ID"=w204) -> ("error out"=w211:errorcluster, "Value"=→"C EB 1":dbl, "Session ID out"=w206:T4)  [unwired: 5 in, 1 out]
                n46 = call <vilib>:"Close Session.vi"("error in (no error)"=w211, "Session ID"=w206) -> ()  [unwired: 9 in, 1 out]
              }
              frame #1 {
                n47 = call <vilib>:"New Session.vi"("Path to Python Module (.py File)"=path "C:/Users/User/Documents/LabVIEW Data/2015 Projects/Combined/Conor_MD_Amb_2models_Buzzi_LabVIEW.py") -> ("error out"=w250:errorcluster, "Session ID out"=w249:T4)  [unwired: 9 in]
                n48 = call <vilib>:"Pack.vi"("Argument"=w214, "error in (no error)"=w250, "Session ID"=w249) -> ("error out"=w243:errorcluster, "Python Object References Out"=w244:T5, "Session ID out"=w245:T4)  [unwired: 6 in]
                n49 = call <vilib>:"Pack.vi"("Argument"=w213, "error in (no error)"=w243, "Python Object References In"=w244, "Session ID"=w245) -> ("error out"=w227:errorcluster, "Python Object References Out"=w229:T5, "Session ID out"=w228:T4)  [unwired: 5 in]
                n50 = call <vilib>:"Pack.vi"("Argument"=w212, "error in (no error)"=w227, "Python Object References In"=w229, "Session ID"=w228) -> ("error out"=w230:errorcluster, "Python Object References Out"=w231:T5, "Session ID out"=w232:T4)  [unwired: 5 in]
                n51 = call <vilib>:"Call.vi"("Function or Method Name"="MD_Buzzi", "error in (no error)"=w230, "Python Object References In"=w231, "Session ID"=w232) -> ("error out"=w236:errorcluster, "Python Object References Out"=w239:T5, "Session ID out"=w242:T4)  [unwired: 5 in]
                n52 = call-poly <vilib>:"Unpack.vi"("error in (no error)"=w236, "Python Object References In"=w239, "Session ID"=w242) -> ("error out"=w223:errorcluster, "Value"=w221:dbl, "Python Object References Out"=w238:T5, "Session ID out"=w241:T4)  [unwired: 5 in]
                "Temp 2" <- w221
                n53 = call-poly <vilib>:"Unpack.vi"("error in (no error)"=w223, "Python Object References In"=w238, "Session ID"=w241) -> ("error out"=w235:errorcluster, "Value"=w220:dbl, "Python Object References Out"=w237:T5, "Session ID out"=w240:T4)  [unwired: 5 in]
                "Flow 2" <- w220
                n54 = call-poly <vilib>:"Unpack.vi"("error in (no error)"=w235, "Python Object References In"=w237, "Session ID"=w240) -> ("error out"=w222:errorcluster, "Value"=w219:dbl, "Python Object References Out"=w233:T5, "Session ID out"=w234:T4)  [unwired: 5 in]
                "Conc 2" <- w219
                n55 = call-poly <vilib>:"Unpack.vi"("error in (no error)"=w222, "Python Object References In"=w233, "Session ID"=w234) -> ("error out"=w255:errorcluster, "Value"=→"X2 A 1":dbl, "Python Object References Out"=w253:T5, "Session ID out"=w251:T4)  [unwired: 5 in]
                n56 = call-poly <vilib>:"Unpack.vi"("error in (no error)"=w255, "Python Object References In"=w253, "Session ID"=w251) -> ("error out"=w256:errorcluster, "Value"=→"X2 ref A 1":dbl, "Python Object References Out"=w254:T5, "Session ID out"=w252:T4)  [unwired: 5 in]
                n57 = call-poly <vilib>:"Unpack.vi"("error in (no error)"=w256, "Python Object References In"=w254, "Session ID"=w252) -> ("error out"=w257:errorcluster, "Value"=→"X2 B 1":dbl, "Python Object References Out"=w248:T5, "Session ID out"=w247:T4)  [unwired: 5 in]
                n58 = call-poly <vilib>:"Unpack.vi"("error in (no error)"=w257, "Python Object References In"=w248, "Session ID"=w247) -> ("error out"=w225:errorcluster, "Value"=→"X ref B 1":dbl, "Session ID out"=w226:T4)  [unwired: 5 in, 1 out]
                n59 = call <vilib>:"Close Session.vi"("error in (no error)"=w225, "Session ID"=w226) -> ()  [unwired: 9 in, 1 out]
              }
            }
            "Exp 2" <- TRUE
          }
          frame 3 {
            n60 = flat-sequence {
              tunnel: w264 -> [w275]
              tunnel: w260 -> [w268]
              tunnel: [w297] -> w263
              tunnel: [w296] -> w262
              tunnel: [w295] -> w261
              tunnel: w260 -> [w290]
              tunnel: w259 -> [w289]
              tunnel: w258 -> [w288]
              frame #0 {
                n61 = call <vilib>:"New Session.vi"("Path to Python Module (.py File)"=path "C:/Users/User/Documents/LabVIEW Data/2015 Projects/Combined/HPLCandAppendAmb.py") -> ("error out"=w284:errorcluster, "Session ID out"=w283:T4)  [unwired: 9 in]
                n62 = call <vilib>:"Pack.vi"("Argument"=w275, "error in (no error)"=w284, "Session ID"=w283) -> ("error out"=w270:errorcluster, "Python Object References Out"=w272:T5, "Session ID out"=w274:T4)  [unwired: 6 in]
                n63 = call <vilib>:"Pack.vi"("Argument"=w268, "error in (no error)"=w270, "Python Object References In"=w272, "Session ID"=w274) -> ("error out"=w269:errorcluster, "Python Object References Out"=w271:T5, "Session ID out"=w273:T4)  [unwired: 5 in]
                n64 = call <vilib>:"Call.vi"("Function or Method Name"="HPLC", "error in (no error)"=w269, "Python Object References In"=w271, "Session ID"=w273) -> ("error out"=w285:errorcluster, "Python Object References Out"=w276:T5, "Session ID out"=w277:T4)  [unwired: 5 in]
                n65 = call-poly <vilib>:"Unpack.vi"("error in (no error)"=w285, "Python Object References In"=w276, "Session ID"=w277) -> ("error out"=w286:errorcluster, "Value"=→"C BAcid 2":dbl, "Python Object References Out"=w281:T5, "Session ID out"=w280:T4)  [unwired: 5 in]
                n66 = call-poly <vilib>:"Unpack.vi"("error in (no error)"=w286, "Python Object References In"=w281, "Session ID"=w280) -> ("error out"=w287:errorcluster, "Value"=→"C EB 2":dbl, "Session ID out"=w282:T4)  [unwired: 5 in, 1 out]
                n67 = call <vilib>:"Close Session.vi"("error in (no error)"=w287, "Session ID"=w282) -> ()  [unwired: 9 in, 1 out]
              }
              frame #1 {
                n68 = call <vilib>:"New Session.vi"("Path to Python Module (.py File)"=path "C:/Users/User/Documents/LabVIEW Data/2015 Projects/Combined/Conor_MD_Amb_2models_Buzzi_LabVIEW.py") -> ("error out"=w326:errorcluster, "Session ID out"=w325:T4)  [unwired: 9 in]
                n69 = call <vilib>:"Pack.vi"("Argument"=w290, "error in (no error)"=w326, "Session ID"=w325) -> ("error out"=w319:errorcluster, "Python Object References Out"=w320:T5, "Session ID out"=w321:T4)  [unwired: 6 in]
                n70 = call <vilib>:"Pack.vi"("Argument"=w289, "error in (no error)"=w319, "Python Object References In"=w320, "Session ID"=w321) -> ("error out"=w303:errorcluster, "Python Object References Out"=w305:T5, "Session ID out"=w304:T4)  [unwired: 5 in]
                n71 = call <vilib>:"Pack.vi"("Argument"=w288, "error in (no error)"=w303, "Python Object References In"=w305, "Session ID"=w304) -> ("error out"=w306:errorcluster, "Python Object References Out"=w307:T5, "Session ID out"=w308:T4)  [unwired: 5 in]
                n72 = call <vilib>:"Call.vi"("Function or Method Name"="MD_Buzzi", "error in (no error)"=w306, "Python Object References In"=w307, "Session ID"=w308) -> ("error out"=w312:errorcluster, "Python Object References Out"=w315:T5, "Session ID out"=w318:T4)  [unwired: 5 in]
                n73 = call-poly <vilib>:"Unpack.vi"("error in (no error)"=w312, "Python Object References In"=w315, "Session ID"=w318) -> ("error out"=w299:errorcluster, "Value"=w297:dbl, "Python Object References Out"=w314:T5, "Session ID out"=w317:T4)  [unwired: 5 in]
                "Temp 3" <- w297
                n74 = call-poly <vilib>:"Unpack.vi"("error in (no error)"=w299, "Python Object References In"=w314, "Session ID"=w317) -> ("error out"=w311:errorcluster, "Value"=w296:dbl, "Python Object References Out"=w313:T5, "Session ID out"=w316:T4)  [unwired: 5 in]
                "Flow 3" <- w296
                n75 = call-poly <vilib>:"Unpack.vi"("error in (no error)"=w311, "Python Object References In"=w313, "Session ID"=w316) -> ("error out"=w298:errorcluster, "Value"=w295:dbl, "Python Object References Out"=w309:T5, "Session ID out"=w310:T4)  [unwired: 5 in]
                "Conc 3" <- w295
                n76 = call-poly <vilib>:"Unpack.vi"("error in (no error)"=w298, "Python Object References In"=w309, "Session ID"=w310) -> ("error out"=w331:errorcluster, "Value"=→"X2 A 2":dbl, "Python Object References Out"=w329:T5, "Session ID out"=w327:T4)  [unwired: 5 in]
                n77 = call-poly <vilib>:"Unpack.vi"("error in (no error)"=w331, "Python Object References In"=w329, "Session ID"=w327) -> ("error out"=w332:errorcluster, "Value"=→"X2 ref A 2":dbl, "Python Object References Out"=w330:T5, "Session ID out"=w328:T4)  [unwired: 5 in]
                n78 = call-poly <vilib>:"Unpack.vi"("error in (no error)"=w332, "Python Object References In"=w330, "Session ID"=w328) -> ("error out"=w333:errorcluster, "Value"=→"X2 B 2":dbl, "Python Object References Out"=w324:T5, "Session ID out"=w323:T4)  [unwired: 5 in]
                n79 = call-poly <vilib>:"Unpack.vi"("error in (no error)"=w333, "Python Object References In"=w324, "Session ID"=w323) -> ("error out"=w301:errorcluster, "Value"=→"X ref B 2":dbl, "Session ID out"=w302:T4)  [unwired: 5 in, 1 out]
                n80 = call <vilib>:"Close Session.vi"("error in (no error)"=w301, "Session ID"=w302) -> ()  [unwired: 9 in, 1 out]
              }
            }
            "Exp 3" <- TRUE
          }
          frame 4 {
            n81 = flat-sequence {
              tunnel: w340 -> [w351]
              tunnel: w336 -> [w344]
              tunnel: [w373] -> w339
              tunnel: [w372] -> w338
              tunnel: [w371] -> w337
              tunnel: w336 -> [w366]
              tunnel: w335 -> [w365]
              tunnel: w334 -> [w364]
              frame #0 {
                n82 = call <vilib>:"New Session.vi"("Path to Python Module (.py File)"=path "C:/Users/User/Documents/LabVIEW Data/2015 Projects/Combined/HPLCandAppendAmb.py") -> ("error out"=w360:errorcluster, "Session ID out"=w359:T4)  [unwired: 9 in]
                n83 = call <vilib>:"Pack.vi"("Argument"=w351, "error in (no error)"=w360, "Session ID"=w359) -> ("error out"=w346:errorcluster, "Python Object References Out"=w348:T5, "Session ID out"=w350:T4)  [unwired: 6 in]
                n84 = call <vilib>:"Pack.vi"("Argument"=w344, "error in (no error)"=w346, "Python Object References In"=w348, "Session ID"=w350) -> ("error out"=w345:errorcluster, "Python Object References Out"=w347:T5, "Session ID out"=w349:T4)  [unwired: 5 in]
                n85 = call <vilib>:"Call.vi"("Function or Method Name"="HPLC", "error in (no error)"=w345, "Python Object References In"=w347, "Session ID"=w349) -> ("error out"=w361:errorcluster, "Python Object References Out"=w352:T5, "Session ID out"=w353:T4)  [unwired: 5 in]
                n86 = call-poly <vilib>:"Unpack.vi"("error in (no error)"=w361, "Python Object References In"=w352, "Session ID"=w353) -> ("error out"=w362:errorcluster, "Value"=→"C BAcid 3":dbl, "Python Object References Out"=w357:T5, "Session ID out"=w356:T4)  [unwired: 5 in]
                n87 = call-poly <vilib>:"Unpack.vi"("error in (no error)"=w362, "Python Object References In"=w357, "Session ID"=w356) -> ("error out"=w363:errorcluster, "Value"=→"C EB 3":dbl, "Session ID out"=w358:T4)  [unwired: 5 in, 1 out]
                n88 = call <vilib>:"Close Session.vi"("error in (no error)"=w363, "Session ID"=w358) -> ()  [unwired: 9 in, 1 out]
              }
              frame #1 {
                n89 = call <vilib>:"New Session.vi"("Path to Python Module (.py File)"=path "C:/Users/User/Documents/LabVIEW Data/2015 Projects/Combined/Conor_MD_Amb_2models_Buzzi_LabVIEW.py") -> ("error out"=w402:errorcluster, "Session ID out"=w401:T4)  [unwired: 9 in]
                n90 = call <vilib>:"Pack.vi"("Argument"=w366, "error in (no error)"=w402, "Session ID"=w401) -> ("error out"=w395:errorcluster, "Python Object References Out"=w396:T5, "Session ID out"=w397:T4)  [unwired: 6 in]
                n91 = call <vilib>:"Pack.vi"("Argument"=w365, "error in (no error)"=w395, "Python Object References In"=w396, "Session ID"=w397) -> ("error out"=w379:errorcluster, "Python Object References Out"=w381:T5, "Session ID out"=w380:T4)  [unwired: 5 in]
                n92 = call <vilib>:"Pack.vi"("Argument"=w364, "error in (no error)"=w379, "Python Object References In"=w381, "Session ID"=w380) -> ("error out"=w382:errorcluster, "Python Object References Out"=w383:T5, "Session ID out"=w384:T4)  [unwired: 5 in]
                n93 = call <vilib>:"Call.vi"("Function or Method Name"="MD_Buzzi", "error in (no error)"=w382, "Python Object References In"=w383, "Session ID"=w384) -> ("error out"=w388:errorcluster, "Python Object References Out"=w391:T5, "Session ID out"=w394:T4)  [unwired: 5 in]
                n94 = call-poly <vilib>:"Unpack.vi"("error in (no error)"=w388, "Python Object References In"=w391, "Session ID"=w394) -> ("error out"=w375:errorcluster, "Value"=w373:dbl, "Python Object References Out"=w390:T5, "Session ID out"=w393:T4)  [unwired: 5 in]
                "Temp 4" <- w373
                n95 = call-poly <vilib>:"Unpack.vi"("error in (no error)"=w375, "Python Object References In"=w390, "Session ID"=w393) -> ("error out"=w387:errorcluster, "Value"=w372:dbl, "Python Object References Out"=w389:T5, "Session ID out"=w392:T4)  [unwired: 5 in]
                "Flow 4" <- w372
                n96 = call-poly <vilib>:"Unpack.vi"("error in (no error)"=w387, "Python Object References In"=w389, "Session ID"=w392) -> ("error out"=w374:errorcluster, "Value"=w371:dbl, "Python Object References Out"=w385:T5, "Session ID out"=w386:T4)  [unwired: 5 in]
                "Conc 4" <- w371
                n97 = call-poly <vilib>:"Unpack.vi"("error in (no error)"=w374, "Python Object References In"=w385, "Session ID"=w386) -> ("error out"=w407:errorcluster, "Value"=→"X2 A 3":dbl, "Python Object References Out"=w405:T5, "Session ID out"=w403:T4)  [unwired: 5 in]
                n98 = call-poly <vilib>:"Unpack.vi"("error in (no error)"=w407, "Python Object References In"=w405, "Session ID"=w403) -> ("error out"=w408:errorcluster, "Value"=→"X2 ref A 3":dbl, "Python Object References Out"=w406:T5, "Session ID out"=w404:T4)  [unwired: 5 in]
                n99 = call-poly <vilib>:"Unpack.vi"("error in (no error)"=w408, "Python Object References In"=w406, "Session ID"=w404) -> ("error out"=w409:errorcluster, "Value"=→"X2 B 3":dbl, "Python Object References Out"=w400:T5, "Session ID out"=w399:T4)  [unwired: 5 in]
                n100 = call-poly <vilib>:"Unpack.vi"("error in (no error)"=w409, "Python Object References In"=w400, "Session ID"=w399) -> ("error out"=w377:errorcluster, "Value"=→"X ref B 3":dbl, "Session ID out"=w378:T4)  [unwired: 5 in, 1 out]
                n101 = call <vilib>:"Close Session.vi"("error in (no error)"=w377, "Session ID"=w378) -> ()  [unwired: 9 in, 1 out]
              }
            }
            "Exp 4" <- TRUE
          }
          frame 5 {
            n102 = flat-sequence {
              tunnel: w416 -> [w427]
              tunnel: w412 -> [w420]
              tunnel: [w449] -> w415
              tunnel: [w448] -> w414
              tunnel: [w447] -> w413
              tunnel: w412 -> [w442]
              tunnel: w411 -> [w441]
              tunnel: w410 -> [w440]
              frame #0 {
                n103 = call <vilib>:"New Session.vi"("Path to Python Module (.py File)"=path "C:/Users/User/Documents/LabVIEW Data/2015 Projects/Combined/HPLCandAppendAmb.py") -> ("error out"=w436:errorcluster, "Session ID out"=w435:T4)  [unwired: 9 in]
                n104 = call <vilib>:"Pack.vi"("Argument"=w427, "error in (no error)"=w436, "Session ID"=w435) -> ("error out"=w422:errorcluster, "Python Object References Out"=w424:T5, "Session ID out"=w426:T4)  [unwired: 6 in]
                n105 = call <vilib>:"Pack.vi"("Argument"=w420, "error in (no error)"=w422, "Python Object References In"=w424, "Session ID"=w426) -> ("error out"=w421:errorcluster, "Python Object References Out"=w423:T5, "Session ID out"=w425:T4)  [unwired: 5 in]
                n106 = call <vilib>:"Call.vi"("Function or Method Name"="HPLC", "error in (no error)"=w421, "Python Object References In"=w423, "Session ID"=w425) -> ("error out"=w437:errorcluster, "Python Object References Out"=w428:T5, "Session ID out"=w429:T4)  [unwired: 5 in]
                n107 = call-poly <vilib>:"Unpack.vi"("error in (no error)"=w437, "Python Object References In"=w428, "Session ID"=w429) -> ("error out"=w438:errorcluster, "Value"=→"C BAcid 4":dbl, "Python Object References Out"=w433:T5, "Session ID out"=w432:T4)  [unwired: 5 in]
                n108 = call-poly <vilib>:"Unpack.vi"("error in (no error)"=w438, "Python Object References In"=w433, "Session ID"=w432) -> ("error out"=w439:errorcluster, "Value"=→"C EB 4":dbl, "Session ID out"=w434:T4)  [unwired: 5 in, 1 out]
                n109 = call <vilib>:"Close Session.vi"("error in (no error)"=w439, "Session ID"=w434) -> ()  [unwired: 9 in, 1 out]
              }
              frame #1 {
                n110 = call <vilib>:"New Session.vi"("Path to Python Module (.py File)"=path "C:/Users/User/Documents/LabVIEW Data/2015 Projects/Combined/Conor_MD_Amb_2models_Buzzi_LabVIEW.py") -> ("error out"=w478:errorcluster, "Session ID out"=w477:T4)  [unwired: 9 in]
                n111 = call <vilib>:"Pack.vi"("Argument"=w442, "error in (no error)"=w478, "Session ID"=w477) -> ("error out"=w471:errorcluster, "Python Object References Out"=w472:T5, "Session ID out"=w473:T4)  [unwired: 6 in]
                n112 = call <vilib>:"Pack.vi"("Argument"=w441, "error in (no error)"=w471, "Python Object References In"=w472, "Session ID"=w473) -> ("error out"=w455:errorcluster, "Python Object References Out"=w457:T5, "Session ID out"=w456:T4)  [unwired: 5 in]
                n113 = call <vilib>:"Pack.vi"("Argument"=w440, "error in (no error)"=w455, "Python Object References In"=w457, "Session ID"=w456) -> ("error out"=w458:errorcluster, "Python Object References Out"=w459:T5, "Session ID out"=w460:T4)  [unwired: 5 in]
                n114 = call <vilib>:"Call.vi"("Function or Method Name"="MD_Buzzi", "error in (no error)"=w458, "Python Object References In"=w459, "Session ID"=w460) -> ("error out"=w464:errorcluster, "Python Object References Out"=w467:T5, "Session ID out"=w470:T4)  [unwired: 5 in]
                n115 = call-poly <vilib>:"Unpack.vi"("error in (no error)"=w464, "Python Object References In"=w467, "Session ID"=w470) -> ("error out"=w451:errorcluster, "Value"=w449:dbl, "Python Object References Out"=w466:T5, "Session ID out"=w469:T4)  [unwired: 5 in]
                "Temp 5" <- w449
                n116 = call-poly <vilib>:"Unpack.vi"("error in (no error)"=w451, "Python Object References In"=w466, "Session ID"=w469) -> ("error out"=w463:errorcluster, "Value"=w448:dbl, "Python Object References Out"=w465:T5, "Session ID out"=w468:T4)  [unwired: 5 in]
                "Flow 5" <- w448
                n117 = call-poly <vilib>:"Unpack.vi"("error in (no error)"=w463, "Python Object References In"=w465, "Session ID"=w468) -> ("error out"=w450:errorcluster, "Value"=w447:dbl, "Python Object References Out"=w461:T5, "Session ID out"=w462:T4)  [unwired: 5 in]
                "Conc 5" <- w447
                n118 = call-poly <vilib>:"Unpack.vi"("error in (no error)"=w450, "Python Object References In"=w461, "Session ID"=w462) -> ("error out"=w483:errorcluster, "Value"=→"X2 A 4":dbl, "Python Object References Out"=w481:T5, "Session ID out"=w479:T4)  [unwired: 5 in]
                n119 = call-poly <vilib>:"Unpack.vi"("error in (no error)"=w483, "Python Object References In"=w481, "Session ID"=w479) -> ("error out"=w484:errorcluster, "Value"=→"X2 ref A 4":dbl, "Python Object References Out"=w482:T5, "Session ID out"=w480:T4)  [unwired: 5 in]
                n120 = call-poly <vilib>:"Unpack.vi"("error in (no error)"=w484, "Python Object References In"=w482, "Session ID"=w480) -> ("error out"=w485:errorcluster, "Value"=→"X2 B 4":dbl, "Python Object References Out"=w476:T5, "Session ID out"=w475:T4)  [unwired: 5 in]
                n121 = call-poly <vilib>:"Unpack.vi"("error in (no error)"=w485, "Python Object References In"=w476, "Session ID"=w475) -> ("error out"=w453:errorcluster, "Value"=→"X ref B 4":dbl, "Session ID out"=w454:T4)  [unwired: 5 in, 1 out]
                n122 = call <vilib>:"Close Session.vi"("error in (no error)"=w453, "Session ID"=w454) -> ()  [unwired: 9 in, 1 out]
              }
            }
            "Exp 5" <- TRUE
          }
          frame 6 {
            n123 = flat-sequence {
              tunnel: w492 -> [w503]
              tunnel: w488 -> [w496]
              tunnel: [w525] -> w491
              tunnel: [w524] -> w490
              tunnel: [w523] -> w489
              tunnel: w488 -> [w518]
              tunnel: w487 -> [w517]
              tunnel: w486 -> [w516]
              frame #0 {
                n124 = call <vilib>:"New Session.vi"("Path to Python Module (.py File)"=path "C:/Users/User/Documents/LabVIEW Data/2015 Projects/Combined/HPLCandAppendAmb.py") -> ("error out"=w512:errorcluster, "Session ID out"=w511:T4)  [unwired: 9 in]
                n125 = call <vilib>:"Pack.vi"("Argument"=w503, "error in (no error)"=w512, "Session ID"=w511) -> ("error out"=w498:errorcluster, "Python Object References Out"=w500:T5, "Session ID out"=w502:T4)  [unwired: 6 in]
                n126 = call <vilib>:"Pack.vi"("Argument"=w496, "error in (no error)"=w498, "Python Object References In"=w500, "Session ID"=w502) -> ("error out"=w497:errorcluster, "Python Object References Out"=w499:T5, "Session ID out"=w501:T4)  [unwired: 5 in]
                n127 = call <vilib>:"Call.vi"("Function or Method Name"="HPLC", "error in (no error)"=w497, "Python Object References In"=w499, "Session ID"=w501) -> ("error out"=w513:errorcluster, "Python Object References Out"=w504:T5, "Session ID out"=w505:T4)  [unwired: 5 in]
                n128 = call-poly <vilib>:"Unpack.vi"("error in (no error)"=w513, "Python Object References In"=w504, "Session ID"=w505) -> ("error out"=w514:errorcluster, "Value"=→"C BAcid 5":dbl, "Python Object References Out"=w509:T5, "Session ID out"=w508:T4)  [unwired: 5 in]
                n129 = call-poly <vilib>:"Unpack.vi"("error in (no error)"=w514, "Python Object References In"=w509, "Session ID"=w508) -> ("error out"=w515:errorcluster, "Value"=→"C EB 5":dbl, "Session ID out"=w510:T4)  [unwired: 5 in, 1 out]
                n130 = call <vilib>:"Close Session.vi"("error in (no error)"=w515, "Session ID"=w510) -> ()  [unwired: 9 in, 1 out]
              }
              frame #1 {
                n131 = call <vilib>:"New Session.vi"("Path to Python Module (.py File)"=path "C:/Users/User/Documents/LabVIEW Data/2015 Projects/Combined/Conor_MD_Amb_2models_Buzzi_LabVIEW.py") -> ("error out"=w554:errorcluster, "Session ID out"=w553:T4)  [unwired: 9 in]
                n132 = call <vilib>:"Pack.vi"("Argument"=w518, "error in (no error)"=w554, "Session ID"=w553) -> ("error out"=w547:errorcluster, "Python Object References Out"=w548:T5, "Session ID out"=w549:T4)  [unwired: 6 in]
                n133 = call <vilib>:"Pack.vi"("Argument"=w517, "error in (no error)"=w547, "Python Object References In"=w548, "Session ID"=w549) -> ("error out"=w531:errorcluster, "Python Object References Out"=w533:T5, "Session ID out"=w532:T4)  [unwired: 5 in]
                n134 = call <vilib>:"Pack.vi"("Argument"=w516, "error in (no error)"=w531, "Python Object References In"=w533, "Session ID"=w532) -> ("error out"=w534:errorcluster, "Python Object References Out"=w535:T5, "Session ID out"=w536:T4)  [unwired: 5 in]
                n135 = call <vilib>:"Call.vi"("Function or Method Name"="MD_Buzzi", "error in (no error)"=w534, "Python Object References In"=w535, "Session ID"=w536) -> ("error out"=w540:errorcluster, "Python Object References Out"=w543:T5, "Session ID out"=w546:T4)  [unwired: 5 in]
                n136 = call-poly <vilib>:"Unpack.vi"("error in (no error)"=w540, "Python Object References In"=w543, "Session ID"=w546) -> ("error out"=w527:errorcluster, "Value"=w525:dbl, "Python Object References Out"=w542:T5, "Session ID out"=w545:T4)  [unwired: 5 in]
                "Temp 6" <- w525
                n137 = call-poly <vilib>:"Unpack.vi"("error in (no error)"=w527, "Python Object References In"=w542, "Session ID"=w545) -> ("error out"=w539:errorcluster, "Value"=w524:dbl, "Python Object References Out"=w541:T5, "Session ID out"=w544:T4)  [unwired: 5 in]
                "Flow 6" <- w524
                n138 = call-poly <vilib>:"Unpack.vi"("error in (no error)"=w539, "Python Object References In"=w541, "Session ID"=w544) -> ("error out"=w526:errorcluster, "Value"=w523:dbl, "Python Object References Out"=w537:T5, "Session ID out"=w538:T4)  [unwired: 5 in]
                "Conc 6" <- w523
                n139 = call-poly <vilib>:"Unpack.vi"("error in (no error)"=w526, "Python Object References In"=w537, "Session ID"=w538) -> ("error out"=w559:errorcluster, "Value"=→"X2 A 5":dbl, "Python Object References Out"=w557:T5, "Session ID out"=w555:T4)  [unwired: 5 in]
                n140 = call-poly <vilib>:"Unpack.vi"("error in (no error)"=w559, "Python Object References In"=w557, "Session ID"=w555) -> ("error out"=w560:errorcluster, "Value"=→"X2 ref A 5":dbl, "Python Object References Out"=w558:T5, "Session ID out"=w556:T4)  [unwired: 5 in]
                n141 = call-poly <vilib>:"Unpack.vi"("error in (no error)"=w560, "Python Object References In"=w558, "Session ID"=w556) -> ("error out"=w561:errorcluster, "Value"=→"X2 B 5":dbl, "Python Object References Out"=w552:T5, "Session ID out"=w551:T4)  [unwired: 5 in]
                n142 = call-poly <vilib>:"Unpack.vi"("error in (no error)"=w561, "Python Object References In"=w552, "Session ID"=w551) -> ("error out"=w529:errorcluster, "Value"=→"X ref B 5":dbl, "Session ID out"=w530:T4)  [unwired: 5 in, 1 out]
                n143 = call <vilib>:"Close Session.vi"("error in (no error)"=w529, "Session ID"=w530) -> ()  [unwired: 9 in, 1 out]
              }
            }
            "Exp 6" <- TRUE
          }
          frame 7 {
            n144 = flat-sequence {
              tunnel: w568 -> [w579]
              tunnel: w564 -> [w572]
              tunnel: [w601] -> w567
              tunnel: [w600] -> w566
              tunnel: [w599] -> w565
              tunnel: w564 -> [w594]
              tunnel: w563 -> [w593]
              tunnel: w562 -> [w592]
              frame #0 {
                n145 = call <vilib>:"New Session.vi"("Path to Python Module (.py File)"=path "C:/Users/User/Documents/LabVIEW Data/2015 Projects/Combined/HPLCandAppendAmb.py") -> ("error out"=w588:errorcluster, "Session ID out"=w587:T4)  [unwired: 9 in]
                n146 = call <vilib>:"Pack.vi"("Argument"=w579, "error in (no error)"=w588, "Session ID"=w587) -> ("error out"=w574:errorcluster, "Python Object References Out"=w576:T5, "Session ID out"=w578:T4)  [unwired: 6 in]
                n147 = call <vilib>:"Pack.vi"("Argument"=w572, "error in (no error)"=w574, "Python Object References In"=w576, "Session ID"=w578) -> ("error out"=w573:errorcluster, "Python Object References Out"=w575:T5, "Session ID out"=w577:T4)  [unwired: 5 in]
                n148 = call <vilib>:"Call.vi"("Function or Method Name"="HPLC", "error in (no error)"=w573, "Python Object References In"=w575, "Session ID"=w577) -> ("error out"=w589:errorcluster, "Python Object References Out"=w580:T5, "Session ID out"=w581:T4)  [unwired: 5 in]
                n149 = call-poly <vilib>:"Unpack.vi"("error in (no error)"=w589, "Python Object References In"=w580, "Session ID"=w581) -> ("error out"=w590:errorcluster, "Value"=→"C BAcid 6":dbl, "Python Object References Out"=w585:T5, "Session ID out"=w584:T4)  [unwired: 5 in]
                n150 = call-poly <vilib>:"Unpack.vi"("error in (no error)"=w590, "Python Object References In"=w585, "Session ID"=w584) -> ("error out"=w591:errorcluster, "Value"=→"C EB 6":dbl, "Session ID out"=w586:T4)  [unwired: 5 in, 1 out]
                n151 = call <vilib>:"Close Session.vi"("error in (no error)"=w591, "Session ID"=w586) -> ()  [unwired: 9 in, 1 out]
              }
              frame #1 {
                n152 = call <vilib>:"New Session.vi"("Path to Python Module (.py File)"=path "C:/Users/User/Documents/LabVIEW Data/2015 Projects/Combined/Conor_MD_Amb_2models_Buzzi_LabVIEW.py") -> ("error out"=w630:errorcluster, "Session ID out"=w629:T4)  [unwired: 9 in]
                n153 = call <vilib>:"Pack.vi"("Argument"=w594, "error in (no error)"=w630, "Session ID"=w629) -> ("error out"=w623:errorcluster, "Python Object References Out"=w624:T5, "Session ID out"=w625:T4)  [unwired: 6 in]
                n154 = call <vilib>:"Pack.vi"("Argument"=w593, "error in (no error)"=w623, "Python Object References In"=w624, "Session ID"=w625) -> ("error out"=w607:errorcluster, "Python Object References Out"=w609:T5, "Session ID out"=w608:T4)  [unwired: 5 in]
                n155 = call <vilib>:"Pack.vi"("Argument"=w592, "error in (no error)"=w607, "Python Object References In"=w609, "Session ID"=w608) -> ("error out"=w610:errorcluster, "Python Object References Out"=w611:T5, "Session ID out"=w612:T4)  [unwired: 5 in]
                n156 = call <vilib>:"Call.vi"("Function or Method Name"="MD_Buzzi", "error in (no error)"=w610, "Python Object References In"=w611, "Session ID"=w612) -> ("error out"=w616:errorcluster, "Python Object References Out"=w619:T5, "Session ID out"=w622:T4)  [unwired: 5 in]
                n157 = call-poly <vilib>:"Unpack.vi"("error in (no error)"=w616, "Python Object References In"=w619, "Session ID"=w622) -> ("error out"=w603:errorcluster, "Value"=w601:dbl, "Python Object References Out"=w618:T5, "Session ID out"=w621:T4)  [unwired: 5 in]
                "Temp 7" <- w601
                n158 = call-poly <vilib>:"Unpack.vi"("error in (no error)"=w603, "Python Object References In"=w618, "Session ID"=w621) -> ("error out"=w615:errorcluster, "Value"=w600:dbl, "Python Object References Out"=w617:T5, "Session ID out"=w620:T4)  [unwired: 5 in]
                "Flow 7" <- w600
                n159 = call-poly <vilib>:"Unpack.vi"("error in (no error)"=w615, "Python Object References In"=w617, "Session ID"=w620) -> ("error out"=w602:errorcluster, "Value"=w599:dbl, "Python Object References Out"=w613:T5, "Session ID out"=w614:T4)  [unwired: 5 in]
                "Conc 7" <- w599
                n160 = call-poly <vilib>:"Unpack.vi"("error in (no error)"=w602, "Python Object References In"=w613, "Session ID"=w614) -> ("error out"=w635:errorcluster, "Value"=→"X2 A 6":dbl, "Python Object References Out"=w633:T5, "Session ID out"=w631:T4)  [unwired: 5 in]
                n161 = call-poly <vilib>:"Unpack.vi"("error in (no error)"=w635, "Python Object References In"=w633, "Session ID"=w631) -> ("error out"=w636:errorcluster, "Value"=→"X2 ref A 6":dbl, "Python Object References Out"=w634:T5, "Session ID out"=w632:T4)  [unwired: 5 in]
                n162 = call-poly <vilib>:"Unpack.vi"("error in (no error)"=w636, "Python Object References In"=w634, "Session ID"=w632) -> ("error out"=w637:errorcluster, "Value"=→"X2 B 6":dbl, "Python Object References Out"=w628:T5, "Session ID out"=w627:T4)  [unwired: 5 in]
                n163 = call-poly <vilib>:"Unpack.vi"("error in (no error)"=w637, "Python Object References In"=w628, "Session ID"=w627) -> ("error out"=w605:errorcluster, "Value"=→"X ref B 6":dbl, "Session ID out"=w606:T4)  [unwired: 5 in, 1 out]
                n164 = call <vilib>:"Close Session.vi"("error in (no error)"=w605, "Session ID"=w606) -> ()  [unwired: 9 in, 1 out]
              }
            }
            "Exp 7" <- TRUE
          }
          frame 8 {
            n165 = flat-sequence {
              tunnel: w644 -> [w655]
              tunnel: w640 -> [w648]
              tunnel: [w677] -> w643
              tunnel: [w676] -> w642
              tunnel: [w675] -> w641
              tunnel: w640 -> [w670]
              tunnel: w639 -> [w669]
              tunnel: w638 -> [w668]
              frame #0 {
                n166 = call <vilib>:"New Session.vi"("Path to Python Module (.py File)"=path "C:/Users/User/Documents/LabVIEW Data/2015 Projects/Combined/HPLCandAppendAmb.py") -> ("error out"=w664:errorcluster, "Session ID out"=w663:T4)  [unwired: 9 in]
                n167 = call <vilib>:"Pack.vi"("Argument"=w655, "error in (no error)"=w664, "Session ID"=w663) -> ("error out"=w650:errorcluster, "Python Object References Out"=w652:T5, "Session ID out"=w654:T4)  [unwired: 6 in]
                n168 = call <vilib>:"Pack.vi"("Argument"=w648, "error in (no error)"=w650, "Python Object References In"=w652, "Session ID"=w654) -> ("error out"=w649:errorcluster, "Python Object References Out"=w651:T5, "Session ID out"=w653:T4)  [unwired: 5 in]
                n169 = call <vilib>:"Call.vi"("Function or Method Name"="HPLC", "error in (no error)"=w649, "Python Object References In"=w651, "Session ID"=w653) -> ("error out"=w665:errorcluster, "Python Object References Out"=w656:T5, "Session ID out"=w657:T4)  [unwired: 5 in]
                n170 = call-poly <vilib>:"Unpack.vi"("error in (no error)"=w665, "Python Object References In"=w656, "Session ID"=w657) -> ("error out"=w666:errorcluster, "Value"=→"C BAcid 7":dbl, "Python Object References Out"=w661:T5, "Session ID out"=w660:T4)  [unwired: 5 in]
                n171 = call-poly <vilib>:"Unpack.vi"("error in (no error)"=w666, "Python Object References In"=w661, "Session ID"=w660) -> ("error out"=w667:errorcluster, "Value"=→"C EB 7":dbl, "Session ID out"=w662:T4)  [unwired: 5 in, 1 out]
                n172 = call <vilib>:"Close Session.vi"("error in (no error)"=w667, "Session ID"=w662) -> ()  [unwired: 9 in, 1 out]
              }
              frame #1 {
                n173 = call <vilib>:"New Session.vi"("Path to Python Module (.py File)"=path "C:/Users/User/Documents/LabVIEW Data/2015 Projects/Combined/Conor_MD_Amb_2models_Buzzi_LabVIEW.py") -> ("error out"=w706:errorcluster, "Session ID out"=w705:T4)  [unwired: 9 in]
                n174 = call <vilib>:"Pack.vi"("Argument"=w670, "error in (no error)"=w706, "Session ID"=w705) -> ("error out"=w699:errorcluster, "Python Object References Out"=w700:T5, "Session ID out"=w701:T4)  [unwired: 6 in]
                n175 = call <vilib>:"Pack.vi"("Argument"=w669, "error in (no error)"=w699, "Python Object References In"=w700, "Session ID"=w701) -> ("error out"=w683:errorcluster, "Python Object References Out"=w685:T5, "Session ID out"=w684:T4)  [unwired: 5 in]
                n176 = call <vilib>:"Pack.vi"("Argument"=w668, "error in (no error)"=w683, "Python Object References In"=w685, "Session ID"=w684) -> ("error out"=w686:errorcluster, "Python Object References Out"=w687:T5, "Session ID out"=w688:T4)  [unwired: 5 in]
                n177 = call <vilib>:"Call.vi"("Function or Method Name"="MD_Buzzi", "error in (no error)"=w686, "Python Object References In"=w687, "Session ID"=w688) -> ("error out"=w692:errorcluster, "Python Object References Out"=w695:T5, "Session ID out"=w698:T4)  [unwired: 5 in]
                n178 = call-poly <vilib>:"Unpack.vi"("error in (no error)"=w692, "Python Object References In"=w695, "Session ID"=w698) -> ("error out"=w679:errorcluster, "Value"=w677:dbl, "Python Object References Out"=w694:T5, "Session ID out"=w697:T4)  [unwired: 5 in]
                "Temp 8" <- w677
                n179 = call-poly <vilib>:"Unpack.vi"("error in (no error)"=w679, "Python Object References In"=w694, "Session ID"=w697) -> ("error out"=w691:errorcluster, "Value"=w676:dbl, "Python Object References Out"=w693:T5, "Session ID out"=w696:T4)  [unwired: 5 in]
                "Flow 8" <- w676
                n180 = call-poly <vilib>:"Unpack.vi"("error in (no error)"=w691, "Python Object References In"=w693, "Session ID"=w696) -> ("error out"=w678:errorcluster, "Value"=w675:dbl, "Python Object References Out"=w689:T5, "Session ID out"=w690:T4)  [unwired: 5 in]
                "Conc 8" <- w675
                n181 = call-poly <vilib>:"Unpack.vi"("error in (no error)"=w678, "Python Object References In"=w689, "Session ID"=w690) -> ("error out"=w711:errorcluster, "Value"=→"X2 A 7":dbl, "Python Object References Out"=w709:T5, "Session ID out"=w707:T4)  [unwired: 5 in]
                n182 = call-poly <vilib>:"Unpack.vi"("error in (no error)"=w711, "Python Object References In"=w709, "Session ID"=w707) -> ("error out"=w712:errorcluster, "Value"=→"X2 ref A 7":dbl, "Python Object References Out"=w710:T5, "Session ID out"=w708:T4)  [unwired: 5 in]
                n183 = call-poly <vilib>:"Unpack.vi"("error in (no error)"=w712, "Python Object References In"=w710, "Session ID"=w708) -> ("error out"=w713:errorcluster, "Value"=→"X2 B 7":dbl, "Python Object References Out"=w704:T5, "Session ID out"=w703:T4)  [unwired: 5 in]
                n184 = call-poly <vilib>:"Unpack.vi"("error in (no error)"=w713, "Python Object References In"=w704, "Session ID"=w703) -> ("error out"=w681:errorcluster, "Value"=→"X ref B 7":dbl, "Session ID out"=w682:T4)  [unwired: 5 in, 1 out]
                n185 = call <vilib>:"Close Session.vi"("error in (no error)"=w681, "Session ID"=w682) -> ()  [unwired: 9 in, 1 out]
              }
            }
            "Exp 8" <- TRUE
          }
          frame 9 {
            n186 = flat-sequence {
              tunnel: w720 -> [w731]
              tunnel: w716 -> [w724]
              tunnel: w716 -> [w746]
              tunnel: w715 -> [w745]
              tunnel: w714 -> [w744]
              frame #0 {
                n187 = call <vilib>:"New Session.vi"("Path to Python Module (.py File)"=path "C:/Users/User/Documents/LabVIEW Data/2015 Projects/Combined/HPLCandAppendAmb.py") -> ("error out"=w740:errorcluster, "Session ID out"=w739:T4)  [unwired: 9 in]
                n188 = call <vilib>:"Pack.vi"("Argument"=w731, "error in (no error)"=w740, "Session ID"=w739) -> ("error out"=w726:errorcluster, "Python Object References Out"=w728:T5, "Session ID out"=w730:T4)  [unwired: 6 in]
                n189 = call <vilib>:"Pack.vi"("Argument"=w724, "error in (no error)"=w726, "Python Object References In"=w728, "Session ID"=w730) -> ("error out"=w725:errorcluster, "Python Object References Out"=w727:T5, "Session ID out"=w729:T4)  [unwired: 5 in]
                n190 = call <vilib>:"Call.vi"("Function or Method Name"="HPLC", "error in (no error)"=w725, "Python Object References In"=w727, "Session ID"=w729) -> ("error out"=w741:errorcluster, "Python Object References Out"=w732:T5, "Session ID out"=w733:T4)  [unwired: 5 in]
                n191 = call-poly <vilib>:"Unpack.vi"("error in (no error)"=w741, "Python Object References In"=w732, "Session ID"=w733) -> ("error out"=w742:errorcluster, "Value"=→"C BAcid 8":dbl, "Python Object References Out"=w737:T5, "Session ID out"=w736:T4)  [unwired: 5 in]
                n192 = call-poly <vilib>:"Unpack.vi"("error in (no error)"=w742, "Python Object References In"=w737, "Session ID"=w736) -> ("error out"=w743:errorcluster, "Value"=→"C EB 8":dbl, "Session ID out"=w738:T4)  [unwired: 5 in, 1 out]
                n193 = call <vilib>:"Close Session.vi"("error in (no error)"=w743, "Session ID"=w738) -> ()  [unwired: 9 in, 1 out]
              }
              frame #1 {
                n194 = call <vilib>:"New Session.vi"("Path to Python Module (.py File)"=path "C:/Users/User/Documents/LabVIEW Data/2015 Projects/Combined/Conor_MD_Amb_2models_Buzzi_LabVIEW.py") -> ("error out"=w782:errorcluster, "Session ID out"=w781:T4)  [unwired: 9 in]
                n195 = call <vilib>:"Pack.vi"("Argument"=w746, "error in (no error)"=w782, "Session ID"=w781) -> ("error out"=w775:errorcluster, "Python Object References Out"=w776:T5, "Session ID out"=w777:T4)  [unwired: 6 in]
                n196 = call <vilib>:"Pack.vi"("Argument"=w745, "error in (no error)"=w775, "Python Object References In"=w776, "Session ID"=w777) -> ("error out"=w759:errorcluster, "Python Object References Out"=w761:T5, "Session ID out"=w760:T4)  [unwired: 5 in]
                n197 = call <vilib>:"Pack.vi"("Argument"=w744, "error in (no error)"=w759, "Python Object References In"=w761, "Session ID"=w760) -> ("error out"=w762:errorcluster, "Python Object References Out"=w763:T5, "Session ID out"=w764:T4)  [unwired: 5 in]
                n198 = call <vilib>:"Call.vi"("Function or Method Name"="MD_Buzzi", "error in (no error)"=w762, "Python Object References In"=w763, "Session ID"=w764) -> ("error out"=w768:errorcluster, "Python Object References Out"=w771:T5, "Session ID out"=w774:T4)  [unwired: 5 in]
                n199 = call-poly <vilib>:"Unpack.vi"("error in (no error)"=w768, "Python Object References In"=w771, "Session ID"=w774) -> ("error out"=w755:errorcluster, "Value"=→"Temp 9":dbl, "Python Object References Out"=w770:T5, "Session ID out"=w773:T4)  [unwired: 5 in]
                n200 = call-poly <vilib>:"Unpack.vi"("error in (no error)"=w755, "Python Object References In"=w770, "Session ID"=w773) -> ("error out"=w767:errorcluster, "Value"=→"Flow 9":dbl, "Python Object References Out"=w769:T5, "Session ID out"=w772:T4)  [unwired: 5 in]
                n201 = call-poly <vilib>:"Unpack.vi"("error in (no error)"=w767, "Python Object References In"=w769, "Session ID"=w772) -> ("error out"=w754:errorcluster, "Value"=→"Conc 9":dbl, "Python Object References Out"=w765:T5, "Session ID out"=w766:T4)  [unwired: 5 in]
                n202 = call-poly <vilib>:"Unpack.vi"("error in (no error)"=w754, "Python Object References In"=w765, "Session ID"=w766) -> ("error out"=w787:errorcluster, "Value"=→"X2 A 8":dbl, "Python Object References Out"=w785:T5, "Session ID out"=w783:T4)  [unwired: 5 in]
                n203 = call-poly <vilib>:"Unpack.vi"("error in (no error)"=w787, "Python Object References In"=w785, "Session ID"=w783) -> ("error out"=w788:errorcluster, "Value"=→"X2 ref A 8":dbl, "Python Object References Out"=w786:T5, "Session ID out"=w784:T4)  [unwired: 5 in]
                n204 = call-poly <vilib>:"Unpack.vi"("error in (no error)"=w788, "Python Object References In"=w786, "Session ID"=w784) -> ("error out"=w789:errorcluster, "Value"=→"X2 B 8":dbl, "Python Object References Out"=w780:T5, "Session ID out"=w779:T4)  [unwired: 5 in]
                n205 = call-poly <vilib>:"Unpack.vi"("error in (no error)"=w789, "Python Object References In"=w780, "Session ID"=w779) -> ("error out"=w757:errorcluster, "Value"=→"X ref B 8":dbl, "Session ID out"=w758:T4)  [unwired: 5 in, 1 out]
                n206 = call <vilib>:"Close Session.vi"("error in (no error)"=w757, "Session ID"=w758) -> ()  [unwired: 9 in, 1 out]
              }
            }
            "Exp 9" <- TRUE
          }
        }
      }
      frame True {
        w790 = 0
      }
    }
    n207 = timed-loop {
      tunnel: w119 -> [w943]
      tunnel: w118 -> [w942]
      tunnel: [w891] -> w117
      tunnel: [w890] -> w116
      timing: w115 -> [_]
      timing-out: [_] -> w114
      tunnel: w113 -> [w877]
      tunnel: w112 -> [w881]
      tunnel: w111 -> [w880]
      tunnel: [w876] -> w110
      tunnel: [w875] -> w109
      tunnel: [w857] -> w108
      tunnel: w99 -> [w872]
      tunnel: w98 -> [w806]
      tunnel: w97 -> [w822]
      tunnel: w107 -> [w861]
      tunnel: w106 -> [w860]
      tunnel: w105 -> [w859]
      tunnel: w104 -> [w858]
      shift-right: [w823] -> _
      shift-left: _ -> [w852]
      tunnel: [w855] -> w103
      tunnel: [w854] -> w102
      tunnel: ["Stop everything"] -> w100
      tunnel: "Automated Experiments or Direct Control" -> [w824]
      tunnel: w91 -> [w817]
      tunnel: w90 -> [w816]
      tunnel: [w815] -> w89
      tunnel: [w814] -> w88
      i -> [w843]
      stop <- w850 stop-if-true
      w794 = 7.5 ("Safety Shut Down Pressure (barg)")
      w873 = 180
      # "in case out of range changes conc to within possible range"
      # "1st 4 flowrates\n5,6 temperatures\n7 pressure (1)\n8 gas (1)"
      # "temperature or syringe or pressure"
      # "We are graphing in barg"
      # "temperature or syringe"
      # "Empty Syringe has level of 50"
      n208 = node-c288() -> ()  [unwired: 1 in, 1 out]
      n209 = call-poly <vilib>:"DAQmx Read.vi"("task/channels in"=w817, "error in"=w816) -> ("task out"=w815:refnum<k21>, "data"=w810:dbl, "error out"=w814:errorcluster)  [unwired: 11 in]
      n210 = Multiply(x=5.1522, y=w810) -> (x*y=w813:dbl)
      n211 = Add(x=-2.6852, y=w813) -> (x+y=w795:dbl)
      "Liquid Inlet Pressure (bar g)" <- w795
      n212 = Greater?(x=w806, y=60) -> (0:w807:bool)
      n213 = Less?(x=w806, y=0) -> (x < y?=w804:bool)
      n214 = case shown="False" w807 {
        tunnel: [w947 1] -> w803
        tunnel: w806 -> [w947 _]
        frame False {
        }
        frame True {
        }
      }
      n215 = case shown="False" w804 {
        tunnel: [w945 1] -> w802
        tunnel: w803 -> [w945 _]
        frame False {
        }
        frame True {
        }
      }
      n216 = for {
        N: 4 -> [_]
        tunnel: w943 -> [w1217] mode=indexing
        tunnel: [w1215] -> w937 mode=indexing
        tunnel: [w1212] -> w932 mode=indexing
        tunnel: [w1211] -> w931 mode=indexing
        tunnel: [w1210] -> w930 mode=indexing
        tunnel: w942 -> [w1209] mode=indexing
        i -> [w1216]
        n217 = call "NCS_GetFlowRateIs.vi"("error in (no error)"=w1209, "dosingunit"=w1216, "device handle in"=w1217) -> ("error out"=w1213:errorcluster, "flowrate is"=w1215:dbl, "device handle out"=w1214:u32)
        n218 = call "NCS_GetSyringeLevelIs.vi"("error in (no error)"=w1213, "dosingunit"=w1216, "device handle in"=w1214) -> ("error out"=w1210:errorcluster, "syringe level is"=w1212:dbl, "device handle out"=w1211:u32)
      }
      n219 = Index Array(array=w932, index=0) -> (element=w847:dbl)
      "Syringe Level 1" <- w847
      n220 = Index Array(array=w932, index=3) -> (element=w844:dbl)
      "Syringe Level 4" <- w844
      n221 = Index Array(array=w932, index=1) -> (element=w846:dbl)
      "Syringe Level 2" <- w846
      n222 = Index Array(array=w932, index=2) -> (element=w845:dbl)
      "Syringe Level 3" <- w845
      n223 = case shown="True" "Shut down in empty?\nLeft off, right on" {
        tunnel: [FALSE w1118] -> w848
        tunnel: w847 -> [_ w1117]
        tunnel: w846 -> [_ w1116]
        tunnel: w845 -> [_ w1115]
        tunnel: w844 -> [_ w1114]
        frame False {
        }
        frame True {
          w1119 = 50
          n224 = Less Or Equal?(x=w1116, y=w1119) -> (x <= y?=w1125:bool)
          n225 = Less Or Equal?(x=w1117, y=w1119) -> (x <= y?=w1120:bool)
          n226 = Less Or Equal?(x=w1115, y=w1119) -> (x <= y?=w1123:bool)
          n227 = Less Or Equal?(x=w1114, y=w1119) -> (x <= y?=w1121:bool)
          n228 = Or(x=w1120, y=w1125) -> (x .or. y?=w1124:bool)
          n229 = Or(x=w1124, y=w1123) -> (x .or. y?=w1122:bool)
          n230 = Or(x=w1122, y=w1121) -> (x .or. y?=w1118:bool)
        }
      }
      n231 = Index Array(array=w937, index=0) -> (element=w834:dbl)
      "Flowrate 1 Low" <- w834
      n232 = Index Array(array=w937, index=3) -> (element=w799:dbl)
      "Flowrate 4 High" <- w799
      n233 = Index Array(array=w937, index=1) -> (element=w833:dbl)
      "Flowrate 2 Low" <- w833
      n234 = Index Array(array=w937, index=2) -> (element=w800:dbl)
      "Flowrate 3 High" <- w800
      n235 = case shown="True" "Clear" {
        tunnel: w852 -> [w1126 _]
        tunnel: [w1126 w1127] -> w851
        frame False {
        }
        frame True {
          n236 = Initialize Array(0, 1) -> (w1127:i32[])
        }
      }
      n237 = call-poly <vilib>:"DAQmx Read.vi"("task/channels in"=w861, "error in"=w860) -> ("task out"=w855:refnum<k21>, "data"=w866:dbl[], "error out"=w854:errorcluster)  [unwired: 11 in]
      n238 = Add(x=w834, y=w833) -> (x+y=w801:dbl)
      n239 = Add(x=w801, y=w800) -> (x+y=w836:dbl)
      n240 = Index Array(array=w866, index=0) -> (element=w864:dbl)
      n241 = Add(x=w836, y=w799) -> (x+y=w835:dbl)
      "Total Flowrate (uL/min)" <- w835
      n242 = Divide(x=w801, y=w835) -> (x/y=w828:dbl)
      n243 = Multiply(x=w864, y=w859) -> (x*y=w865:dbl)
      n244 = Multiply(x="Low Conc", y=w828) -> (x*y=w832:dbl)
      n245 = Add(x=w865, y=w858) -> (x+y=w862:dbl)
      n246 = Add(x=w800, y=w799) -> (x+y=w798:dbl)
      n247 = Divide(x=w798, y=w835) -> (x/y=w829:dbl)
      n248 = Multiply(x="High Conc", y=w829) -> (x*y=w831:dbl)
      n249 = Add(x=w832, y=w831) -> (x+y=→"Feed Concentration (M)":dbl)
      n250 = In Range and Coerce(upper limit="High Conc", x=w822, lower limit="Low Conc") -> (coerced(x)=w819:dbl, In Range?=w821:bool)
      n251 = case shown="False" w821 {
        tunnel: [w950 w952] -> w820
        tunnel: w822 -> [_ w952]
        tunnel: w819 -> [w950 _]
        tunnel: [TRUE FALSE] -> w818
        frame False {
        }
        frame True {
        }
      }
      "Desired Conc Not Possible" <- w818
      n252 = Multiply(x=w862, y=0.0689476) -> (x*y=w809:dbl)
      "Gas Back Pressure (barg)" <- w809
      n253 = case shown="False" w824 {
        tunnel: [w1189 w1190] -> w928
        tunnel: w802 -> [w1183 _]
        tunnel: w820 -> [w1186 _]
        tunnel: "High Conc" -> [w1188 _]
        tunnel: "Low Conc" -> [w1187 _]
        frame False {
          # "h-s/h-l"
          # "s-l/h-l"
          # "high flow"
          # "low flow"
          # "2 syringes each"
          # "h-s"
          # "s-l"
          # "h-l"
          n254 = Subtract(x=w1188, y=w1187) -> (x-y=w1176:dbl)
          n255 = Subtract(x=w1186, y=w1187) -> (x-y=w1185:dbl)
          n256 = Subtract(x=w1188, y=w1186) -> (x-y=w1177:dbl)
          n257 = Divide(x=w1183, y=2) -> (x/y=w1182:dbl)
          n258 = Divide(x=w1177, y=w1176) -> (x/y=w1181:dbl)
          n259 = Divide(x=w1185, y=w1176) -> (x/y=w1180:dbl)
          n260 = Multiply(x=w1182, y=w1181) -> (x*y=w1179:dbl)
          n261 = Multiply(x=w1182, y=w1180) -> (x*y=w1178:dbl)
          n262 = Build Array(w1179, w1179, w1178, w1178) -> (w1189:dbl[])
        }
        frame True {
          n263 = Build Array("Set Flowrate 1", "Set Flowrate 2", "Set Flowrate 3", "Set Flowrate 4") -> (w1190:dbl[])
        }
      }
      n264 = Greater Or Equal?(x=w795, y=w794) -> (x >= y?=w793:bool)
      n265 = Build Array (concatenate)(w851, w809) -> (w823:dbl[])
      "Calculated Pressure" <- w823
      n266 = Greater Or Equal?(x=w809, y=w794) -> (x >= y?=w792:bool)
      n267 = Or(x=w793, y=w792) -> (x .or. y?=w791:bool)
      n268 = case shown="True" w824 {
        tunnel: [w1131 FALSE] -> w826
        tunnel: w843 -> [w1130 _]
        frame False {
          # "changes set points for each new exp"
          n269 = Equal?(x=w1130, y=0) -> (x = y?=w1131:bool)
        }
        frame True {
          # "at end of each exp"
          # "doesnt automatically change set point"
        }
      }
      n270 = Or(x=w826, y="Update Temperature Set Point") -> (x .or. y?=w883:bool)
      n271 = case shown="True" w883 {
        tunnel: w881 -> [w1135 w1143]
        tunnel: w880 -> [w1134 w1142]
        tunnel: [w1135 w1141] -> w879
        tunnel: [w1134 w1140] -> w878
        tunnel: w877 -> [_ w1139]
        tunnel: w824 -> [_ w1137]
        tunnel: w872 -> [_ w1136]
        frame False {
        }
        frame True {
          n272 = case shown="False" w1137 {
            tunnel: [w1144 "Set Point (oC)"] -> w1138
            tunnel: w1136 -> [w1144 _]
            frame False {
            }
            frame True {
            }
          }
          n273 = call "CN7500_Write Set Point Value.vi"("Target Set Point Value"=w1138, "error in (no error)"=w1142, "Controller Number"=w1139, "VISA In"=w1143) -> ("error out"=w1140:errorcluster, "VISA Out"=w1141:refnum<visa-resource-name>)  [unwired: 6 in]
        }
      }
      n274 = Or(x="Generate Flow", y=w826) -> (x .or. y?=w827:bool)
      n275 = case shown="True" w827 {
        tunnel: w931 -> [w1196 w1201]
        tunnel: w930 -> [w1195 w1200]
        tunnel: [w1195 w1199] -> w838
        tunnel: [w1196 w1198] -> w837
        tunnel: w928 -> [_ w1197]
        frame False {
        }
        frame True {
          n276 = for {
            N: 4 -> [_]
            tunnel: w1201 -> [w1208] mode=indexing
            tunnel: w1200 -> [w1207] mode=indexing
            tunnel: [w1206] -> w1199 mode=indexing
            tunnel: [w1205] -> w1198 mode=indexing
            tunnel: w1197 -> [w1203] mode=indexing
            i -> [w1204]
            n277 = call "NCS_GenerateFlow.vi"("error in (no error)"=w1207, "flowrate"=w1203, "dosingunit"=w1204, "device handle in"=w1208) -> ("error out"=w1206:errorcluster, "device handle out"=w1205:u32)
          }
        }
      }
      n278 = call "CN7500_Read Process Value.vi"("error in (no error)"=w878, "Controller Number"=w877, "VISA In"=w879) -> ("error out"=w876:errorcluster, "Set Point Value"=w868:dbl, "Process Value"=w869:dbl, "VISA Out"=w875:refnum<visa-resource-name>)  [unwired: 5 in]
      "Temp Set Point (oC)" <- w868
      "Actual Temp (oC)" <- w869
      n279 = Merge Signals(w869, w868) -> (→"Temperature":dynamicdata)
      n280 = Merge Signals(w834, w833, w800, w799, w869, w868, w809, w795) -> (w889:dynamicdata)
      n281 = Greater Or Equal?(x=w869, y=w873) -> (x >= y?=w871:bool)
      n282 = call "Write To Measurement File"("Signals"=w889) -> ()  [unwired: 16 in, 3 out]
      n283 = Index Array(array=w838, index=0) -> (element=w918:errorcluster)
      n284 = Index Array(array=w837, index=0) -> (element=w919:u32)
      n285 = Index Array(array=w838, index=3) -> (element=w908:errorcluster)
      n286 = Index Array(array=w838, index=2) -> (element=w910:errorcluster)
      n287 = Index Array(array=w838, index=1) -> (element=w912:errorcluster)
      n288 = Index Array(array=w837, index=3) -> (element=w909:u32)
      n289 = Index Array(array=w837, index=2) -> (element=w911:u32)
      n290 = Index Array(array=w837, index=1) -> (element=w913:u32)
      n291 = case shown="False" "Stop Dose 2" {
        tunnel: w913 -> [w1163 w1168]
        tunnel: w912 -> [w1162 w1167]
        tunnel: [w1163 w1166] -> w905
        tunnel: [w1162 w1165] -> w904
        frame False {
        }
        frame True {
          n292 = call "NCS_Stop.vi"("error in (no error)"=w1167, "dosingunit"=1, "device handle in"=w1168) -> ("error out"=w1165:errorcluster, "device handle out"=w1166:u32)
        }
      }
      n293 = case shown="False" "Stop Dose 1" {
        tunnel: w919 -> [w1170 w1175]
        tunnel: w918 -> [w1169 w1174]
        tunnel: [w1170 w1173] -> w907
        tunnel: [w1169 w1172] -> w906
        frame False {
        }
        frame True {
          n294 = call "NCS_Stop.vi"("error in (no error)"=w1174, "dosingunit"=0, "device handle in"=w1175) -> ("error out"=w1172:errorcluster, "device handle out"=w1173:u32)
        }
      }
      n295 = case shown="False" "Stop Dose 3" {
        tunnel: w911 -> [w1156 w1161]
        tunnel: w910 -> [w1155 w1160]
        tunnel: [w1156 w1159] -> w903
        tunnel: [w1155 w1158] -> w902
        frame False {
        }
        frame True {
          n296 = call "NCS_Stop.vi"("error in (no error)"=w1160, "dosingunit"=2, "device handle in"=w1161) -> ("error out"=w1158:errorcluster, "device handle out"=w1159:u32)
        }
      }
      n297 = case shown="False" "Stop Dose 4" {
        tunnel: w909 -> [w1149 w1154]
        tunnel: w908 -> [w1148 w1153]
        tunnel: [w1149 w1152] -> w901
        tunnel: [w1148 w1151] -> w900
        frame False {
        }
        frame True {
          n298 = call "NCS_Stop.vi"("error in (no error)"=w1153, "dosingunit"=3, "device handle in"=w1154) -> ("error out"=w1151:errorcluster, "device handle out"=w1152:u32)
        }
      }
      n299 = case shown="False" "Safety or Emergency Syringe Control" {
        tunnel: w907 -> [w960 w1001]
        tunnel: w906 -> [w956 w1000]
        tunnel: w905 -> [w959 w999]
        tunnel: w904 -> [w955 w998]
        tunnel: w903 -> [w958 w997]
        tunnel: w902 -> [w954 w996]
        tunnel: w901 -> [w957 w995]
        tunnel: w900 -> [w953 w994]
        tunnel: [w960 w971] -> w899
        tunnel: [w959 w970] -> w898
        tunnel: [w958 w969] -> w897
        tunnel: [w957 w968] -> w896
        tunnel: [w955 w967] -> w895
        tunnel: [w954 w966] -> w894
        tunnel: [w953 w965] -> w893
        tunnel: [w956 w961] -> w892
        frame False {
        }
        frame True {
          n300 = case shown="False" "Calibrate 2" {
            tunnel: w999 -> [w1100 w1105]
            tunnel: w998 -> [w1099 w1104]
            tunnel: [w1100 w1103] -> w988
            tunnel: [w1099 w1102] -> w987
            frame False {
            }
            frame True {
              n301 = call "NCS_Calibrate.vi"("error in (no error)"=w1104, "dosingunit"=1, "device handle in"=w1105) -> ("error out"=w1102:errorcluster, "device handle out"=w1103:u32)
            }
          }
          n302 = case shown="False" "Calibrate 3" {
            tunnel: w997 -> [w1093 w1098]
            tunnel: w996 -> [w1092 w1097]
            tunnel: [w1093 w1096] -> w986
            tunnel: [w1092 w1095] -> w985
            frame False {
            }
            frame True {
              n303 = call "NCS_Calibrate.vi"("error in (no error)"=w1097, "dosingunit"=2, "device handle in"=w1098) -> ("error out"=w1095:errorcluster, "device handle out"=w1096:u32)
            }
          }
          n304 = case shown="False" "Calibrate 1" {
            tunnel: w1001 -> [w1107 w1112]
            tunnel: w1000 -> [w1106 w1111]
            tunnel: [w1107 w1110] -> w990
            tunnel: [w1106 w1109] -> w989
            frame False {
            }
            frame True {
              n305 = call "NCS_Calibrate.vi"("error in (no error)"=w1111, "dosingunit"=0, "device handle in"=w1112) -> ("error out"=w1109:errorcluster, "device handle out"=w1110:u32)
            }
          }
          n306 = case shown="False" "Calibrate 4" {
            tunnel: w995 -> [w1086 w1091]
            tunnel: w994 -> [w1085 w1090]
            tunnel: [w1086 w1089] -> w984
            tunnel: [w1085 w1088] -> w983
            frame False {
            }
            frame True {
              n307 = call "NCS_Calibrate.vi"("error in (no error)"=w1090, "dosingunit"=3, "device handle in"=w1091) -> ("error out"=w1088:errorcluster, "device handle out"=w1089:u32)
            }
          }
          n308 = case shown="False" "Empty 2" {
            tunnel: w988 -> [w1066 w1070]
            tunnel: w987 -> [w1065 w1068]
            tunnel: [w1066 w1069] -> w974
            tunnel: [w1065 w1067] -> w975
            frame False {
            }
            frame True {
              w1072 = 1
              n309 = call "NCS_GetFlowRateMax.vi"("error in (no error)"=w1068, "dosingunit"=w1072, "device handle in"=w1070) -> ("error out"=w1073:errorcluster, "flow rate max"=w1071:dbl, "device handle out"=w1074:u32)
              n310 = call "NCS_EmptySyrige.vi"("error in (no error)"=w1073, "flowrate"=w1071, "dosingunit"=w1072, "device handle in"=w1074) -> ("error out"=w1067:errorcluster, "device handle out"=w1069:u32)
            }
          }
          n311 = case shown="False" "Empty 1" {
            tunnel: w990 -> [w1076 w1084]
            tunnel: w989 -> [w1075 w1081]
            tunnel: [w1076 w1082] -> w972
            tunnel: [w1075 w1079] -> w973
            frame False {
            }
            frame True {
              w1078 = 0
              n312 = call "NCS_GetFlowRateMax.vi"("error in (no error)"=w1081, "dosingunit"=w1078, "device handle in"=w1084) -> ("error out"=w1080:errorcluster, "flow rate max"=w1077:dbl, "device handle out"=w1083:u32)
              n313 = call "NCS_EmptySyrige.vi"("error in (no error)"=w1080, "flowrate"=w1077, "dosingunit"=w1078, "device handle in"=w1083) -> ("error out"=w1079:errorcluster, "device handle out"=w1082:u32)
            }
          }
          n314 = case shown="False" "Empty 3" {
            tunnel: w986 -> [w1056 w1057]
            tunnel: w985 -> [w1055 w1058]
            tunnel: [w1056 w1059] -> w976
            tunnel: [w1055 w1060] -> w977
            frame False {
            }
            frame True {
              w1062 = 2
              n315 = call "NCS_GetFlowRateMax.vi"("error in (no error)"=w1058, "dosingunit"=w1062, "device handle in"=w1057) -> ("error out"=w1063:errorcluster, "flow rate max"=w1061:dbl, "device handle out"=w1064:u32)
              n316 = call "NCS_EmptySyrige.vi"("error in (no error)"=w1063, "flowrate"=w1061, "dosingunit"=w1062, "device handle in"=w1064) -> ("error out"=w1060:errorcluster, "device handle out"=w1059:u32)
            }
          }
          n317 = case shown="False" "Empty 4" {
            tunnel: w984 -> [w1046 w1047]
            tunnel: w983 -> [w1045 w1048]
            tunnel: [w1046 w1050] -> w978
            tunnel: [w1045 w1049] -> w979
            frame False {
            }
            frame True {
              w1052 = 3
              n318 = call "NCS_GetFlowRateMax.vi"("error in (no error)"=w1048, "dosingunit"=w1052, "device handle in"=w1047) -> ("error out"=w1053:errorcluster, "flow rate max"=w1051:dbl, "device handle out"=w1054:u32)
              n319 = call "NCS_EmptySyrige.vi"("error in (no error)"=w1053, "flowrate"=w1051, "dosingunit"=w1052, "device handle in"=w1054) -> ("error out"=w1049:errorcluster, "device handle out"=w1050:u32)
            }
          }
          n320 = case shown="False" "Refill 2" {
            tunnel: w974 -> [w1026 w1030]
            tunnel: w975 -> [w1025 w1028]
            tunnel: [w1026 w1029] -> w970
            tunnel: [w1025 w1027] -> w967
            frame False {
            }
            frame True {
              w1032 = 1
              n321 = call "NCS_GetFlowRateMax.vi"("error in (no error)"=w1028, "dosingunit"=w1032, "device handle in"=w1030) -> ("error out"=w1033:errorcluster, "flow rate max"=w1031:dbl, "device handle out"=w1034:u32)
              n322 = call "NCS_RefillSyrige.vi"("error in (no error)"=w1033, "flowrate"=w1031, "dosingunit"=w1032, "device handle in"=w1034) -> ("error out"=w1027:errorcluster, "device handle out"=w1029:u32)
            }
          }
          n323 = case shown="False" "Refill 1" {
            tunnel: w972 -> [w1036 w1044]
            tunnel: w973 -> [w1035 w1041]
            tunnel: [w1036 w1042] -> w971
            tunnel: [w1035 w1039] -> w961
            frame False {
            }
            frame True {
              w1038 = 0
              n324 = call "NCS_GetFlowRateMax.vi"("error in (no error)"=w1041, "dosingunit"=w1038, "device handle in"=w1044) -> ("error out"=w1040:errorcluster, "flow rate max"=w1037:dbl, "device handle out"=w1043:u32)
              n325 = call "NCS_RefillSyrige.vi"("error in (no error)"=w1040, "flowrate"=w1037, "dosingunit"=w1038, "device handle in"=w1043) -> ("error out"=w1039:errorcluster, "device handle out"=w1042:u32)
            }
          }
          n326 = case shown="False" "Refill 3" {
            tunnel: w976 -> [w1016 w1017]
            tunnel: w977 -> [w1015 w1018]
            tunnel: [w1016 w1019] -> w969
            tunnel: [w1015 w1020] -> w966
            frame False {
            }
            frame True {
              w1022 = 2
              n327 = call "NCS_GetFlowRateMax.vi"("error in (no error)"=w1018, "dosingunit"=w1022, "device handle in"=w1017) -> ("error out"=w1023:errorcluster, "flow rate max"=w1021:dbl, "device handle out"=w1024:u32)
              n328 = call "NCS_RefillSyrige.vi"("error in (no error)"=w1023, "flowrate"=w1021, "dosingunit"=w1022, "device handle in"=w1024) -> ("error out"=w1020:errorcluster, "device handle out"=w1019:u32)
            }
          }
          n329 = case shown="False" "Refill 4" {
            tunnel: w978 -> [w1006 w1007]
            tunnel: w979 -> [w1005 w1008]
            tunnel: [w1006 w1010] -> w968
            tunnel: [w1005 w1009] -> w965
            frame False {
            }
            frame True {
              w1012 = 3
              n330 = call "NCS_GetFlowRateMax.vi"("error in (no error)"=w1008, "dosingunit"=w1012, "device handle in"=w1007) -> ("error out"=w1013:errorcluster, "flow rate max"=w1011:dbl, "device handle out"=w1014:u32)
              n331 = call "NCS_RefillSyrige.vi"("error in (no error)"=w1013, "flowrate"=w1011, "dosingunit"=w1012, "device handle in"=w1014) -> ("error out"=w1009:errorcluster, "device handle out"=w1010:u32)
            }
          }
        }
      }
      n332 = Or(x=w871, y=w848) -> (x .or. y?=w856:bool)
      n333 = Or(x=w856, y=w791) -> (x .or. y?=w857:bool)
      n334 = Multiply(x="Minutes between Exp", y=60) -> (x*y=w840:dbl)
      n335 = Divide(x=w840, y=5) -> (x/y=w841:dbl)
      n336 = Greater Or Equal?(x=w843, y=w841) -> (x >= y?=w885:bool)
      n337 = Or(x=w885, y=w857) -> (x .or. y?=w870:bool)
      n338 = Or(x="Skip Exp", y=w870) -> (x .or. y?=w886:bool)
      n339 = Or(x="Stop everything", y=w886) -> (x .or. y?=w850:bool)
      n340 = node-c288() -> ()  [unwired: 1 in, 1 out]
      n341 = Build Array(w899, w898, w897, w896) -> (w891:u32[])
      n342 = Build Array(w892, w895, w894, w893) -> (w890:errorcluster[])
      "loop ind" <- w843
      "Safety Shut Down Temp" <- w873
      "Safety Shut Down Pressure (barg)" <- w794
    }
    n343 = Or(x=w100, y=w108) -> (x .or. y?=w101:bool)
    n344 = node-c288(w114) -> ()  [unwired: 1 out]
    "HPLC file name, MBDoE2peakin1" <- w85
    "Record filename, RecordAmbInitisileFactorial1" <- w84
  }
  n345 = call <vilib>:"DAQmx Stop Task.vi"("task/channels in"=w18, "error in"=w17) -> ("task out"=w20:refnum<k21>, "error out"=w19:errorcluster)  [unwired: 12 in]
  n346 = Index Array(array=w47, index=0) -> (element=w49:u32)
  n347 = Index Array(array=w46, index=0) -> (element=w48:errorcluster)
  n348 = call <vilib>:"DAQmx Stop Task.vi"("task/channels in"=w7, "error in"=w5) -> ("task out"=w6:refnum<k21>, "error out"=w8:errorcluster)  [unwired: 12 in]
  n349 = call <vilib>:"DAQmx Clear Task.vi"("task in"=w20, "error in"=w19) -> ()  [unwired: 13 in, 1 out]
  n350 = call <vilib>:"DAQmx Clear Task.vi"("task in"=w6, "error in"=w8) -> ()  [unwired: 13 in, 1 out]
  n351 = call "NCS_CloseDevice.vi"("error in (no error)"=w48, "device handle"=w49) -> ()  [unwired: 1 out]
  n352 = call "CN7500_Write Set Point Value.vi"("Target Set Point Value"=25, "error in (no error)"=w35, "Controller Number"=w38, "VISA In"=w34) -> ("error out"=w40:errorcluster, "VISA Out"=w41:refnum<visa-resource-name>)  [unwired: 6 in]
  n353 = call "CN7500_Close.vi"("error in (no error)"=w40, "VISA resource name"=w41) -> ()  [unwired: 9 in, 1 out]
